vi "AO_master_DM_WFS_v1_SynModeFailure_discarded.vi"() -> ()   [LabVIEW 2018]
uses:
  <userlib>/WaveKit.lib/Controls/Image information.ctl
  <userlib>/WaveKit.lib/Controls/Image general information.ctl
  <userlib>/WaveKit.lib/Controls/Image acquisition information.ctl
  <userlib>/WaveKit.lib/Controls/Point2D.ctl
  <userlib>/WaveKit.lib/Controls/Data alignment enum.ctl
  <userlib>/WaveKit.lib/Controls/StatisticsData.ctl
  <userlib>/WaveKit.lib/Controls/Wavefront Corrector states - ONE.ctl
  <userlib>/WaveKit.lib/Classes/Camera/Camera.lvclass
  <userlib>/WaveKit.lib/Classes/CameraSet/CameraSet.lvclass
  <userlib>/WaveKit.lib/Classes/Image/Image.lvclass
  <userlib>/WaveKit.lib/Classes/Phase/Phase.lvclass
  <userlib>/WaveKit.lib/Controls/HasoSlopes.lvclass
  <userlib>/WaveKit.lib/Controls/Pupil.lvclass
  <userlib>/WaveKit.lib/Classes/WavefrontCorrector/WavefrontCorrector.lvclass
  <userlib>/WaveKit.lib/Classes/WavefrontCorrectorSet/WavefrontCorrectorSet.lvclass
  <userlib>/WaveKit.lib/Classes/HasoEngine/HasoEngine.lvclass
  <userlib>/WaveKit.lib/Controls/SlopesEngineSetup.ctl
  <userlib>/WaveKit.lib/Controls/WavefrontReconstructionMode.ctl
  <vilib>/Utility/file.llb/Read From Spreadsheet File (DBL).vi
  <vilib>/Analysis/1siggen.llb/Ramp Pattern by Delta.vi
  <userlib>/WaveKit.lib/Classes/ModalCoef/ModalCoef.lvclass
  <vilib>/Analysis/NI_AALBase.lvlib
panel:
  in  "Device Status":enum32{"DM", "WFS", "Others"}(tab)
  out "DM Actuator Values":sgl[](graph)
  out "Initial State":T1[](array[typedef])
  out "ActuatorsNumber":i32
  out "Initial Positions":sgl[](array[numeric])
  out "Final Positions":sgl[](array[numeric])
  in  "Coef Min":dbl=-0.5 min=1.0
  in  "Coef Max":dbl=0.5 min=1.0
  out "Zernike Measured":dbl[](graph)
  out "Phase statistics":T2
  out "Phase values":sgl[][](graph)=[[nan, nan, nan, nan, nan, nan, nan, nan, nan, nan, nan, nan, nan, nan, nan, nan, nan, nan, nan, nan, nan, nan, nan, nan, nan, nan, nan, nan, nan, nan, nan, nan, nan, nan, nan, nan, nan, nan, nan, nan], [nan, nan, nan, nan, nan, nan, nan, nan, nan, nan, nan, nan, nan, nan, nan, nan, nan, nan, nan, nan, nan, nan, nan, nan, nan, nan, nan, nan, nan, nan, nan, nan, nan, nan, nan, nan, nan, nan, nan, nan], [nan, nan, nan, nan, nan, nan, nan, nan, nan, nan, nan, nan, nan, nan, nan, nan, nan, nan, nan, nan, nan, nan, nan, nan, nan, nan, nan, nan, nan, nan, nan, nan, nan, nan, nan, nan, nan, nan, nan, nan], [nan, nan, nan, nan, nan, nan, nan, nan, nan, nan, nan, nan, nan, nan, nan, nan, nan, nan, nan, nan, nan, nan, nan, nan, nan, nan, nan, nan, nan, nan, nan, nan, nan, nan, nan, nan, nan, nan, nan, nan], [nan, nan, nan, nan, nan, nan, nan, nan, nan, nan, nan, nan, nan, nan, -0.14441992, nan, 0.1501734, 0.22490476, 0.2674259, 0.28415325, 0.2792031, 0.2552752, 0.21375881, 0.15405469, nan, nan, nan, nan, nan, nan, nan, nan, nan, nan, nan, nan, nan, nan, nan, nan], [nan, nan, nan, nan, nan, nan, nan, nan, nan, nan, nan, nan, nan, nan, 0.19143742, 0.2795512, 0.33646506, 0.37099743, 0.3877919, 0.3894302, 0.37774685, 0.35447162, 0.3212538, 0.27904776, 0.22675864, 0.15897867, nan, nan, nan, nan, nan, nan, nan, nan, nan, nan, nan, nan, nan, nan], [nan, nan, nan, nan, nan, nan, nan, nan, nan, nan, nan, nan, nan, 0.22618562, 0.290776, 0.33285964, 0.36044422, 0.3767934, 0.38285175, 0.37884915, 0.3652757, 0.3433441, 0.3149789, 0.28229773, 0.2464756, 0.20580466, 0.15268901, 0.06923797, nan, nan, nan, nan, nan, nan, nan, nan, nan, nan, nan, nan], [nan, nan, nan, nan, nan, nan, nan, nan, nan, nan, nan, nan, 0.19992779, 0.24616541, 0.27565512, 0.29675642, 0.31222007, 0.32191983, 0.32467726, 0.31943765, 0.30597392, 0.2852214, 0.25927368, 0.2309889, 0.20308714, 0.17653626, 0.14795627, 0.10568966, 0.024115691, nan, nan, nan, nan, nan, nan, nan, nan, nan, nan, nan], [nan, nan, nan, nan, nan, nan, nan, nan, nan, nan, nan, 0.14862825, 0.18219855, 0.20114602, 0.21551609, 0.22862102, 0.24014233, 0.24817906, 0.2505626, 0.24567793, 0.23295718, 0.21313797, 0.18829979, 0.16161954, 0.1367108, 0.11633411, 0.10019377, 0.081457645, 0.04156301, -0.057204023, nan, nan, nan, nan, nan, nan, nan, nan, nan, nan], [nan, nan, nan, nan, nan, nan, nan, nan, nan, nan, 0.08899155, 0.117771566, 0.12948777, 0.13732892, 0.14631097, 0.15688494, 0.16728252, 0.17497937, 0.17758016, 0.17335457, 0.16157834, 0.14275661, 0.11873307, 0.09261118, 0.06834036, 0.04974218, 0.038678437, 0.031985473, 0.016725859, -0.03676957, nan, nan, nan, nan, nan, nan, nan, nan, nan, nan], [nan, nan, nan, nan, nan, nan, nan, nan, nan, nan, 0.058377307, 0.069048055, 0.0725615, 0.07683456, 0.0840318, 0.09335055, 0.10271386, 0.1097376, 0.11226265, 0.10867052, 0.09812171, 0.08078306, 0.058033932, 0.032565817, 0.008214329, -0.010712444, -0.020921554, -0.022825297, -0.02489755, -0.05023362, -0.14592764, nan, nan, nan, nan, nan, nan, nan, nan, nan], [nan, nan, nan, nan, nan, nan, nan, nan, nan, -0.0018393314, 0.018310271, 0.023098737, 0.024714457, 0.027986258, 0.033823933, 0.041292578, 0.048749834, 0.054400377, 0.056548227, 0.05374936, 0.04499338, 0.029967438, 0.009379062, -0.014759185, -0.03905803, -0.059140373, -0.070816256, -0.0724436, -0.06894927, -0.07806298, -0.1393881, nan, nan, nan, nan, nan, nan, nan, nan, nan], [nan, nan, nan, nan, nan, nan, nan, nan, nan, -0.03322208, -0.017045017, -0.0123043535, -0.010394985, -0.007970343, -0.0042642877, 0.0003761826, 0.005164365, 0.009095938, 0.010986101, 0.009512841, 0.0033822758, -0.008344227, -0.02579559, -0.047820807, -0.071688615, -0.09321856, -0.107681155, -0.11187886, -0.10789668, -0.10908524, -0.14891545, -0.29341945, nan, nan, nan, nan, nan, nan, nan, nan], [nan, nan, nan, nan, nan, nan, nan, nan, nan, nan, -0.043187555, -0.03622458, -0.033755217, -0.03278728, -0.03198469, -0.030707732, -0.028716512, -0.026208155, -0.023933899, -0.023217455, -0.025771504, -0.03328519, -0.04682974, -0.06620631, -0.08943447, -0.1126552, -0.13079928, -0.13944486, -0.13836564, -0.13734597, -0.16491348, -0.2807172, nan, nan, nan, nan, nan, nan, nan, nan], [nan, nan, nan, nan, nan, nan, nan, nan, -0.13038255, -0.08328184, -0.060542934, -0.050779276, -0.048053104, -0.048984695, -0.05126809, -0.053124577, -0.05330209, -0.051303368, -0.04760214, -0.04368073, -0.041799206, -0.04448101, -0.05377527, -0.07043236, -0.09320336, -0.118551016, -0.14113419, -0.15550357, -0.15952203, -0.16009864, -0.18189941, -0.27977645, nan, nan, nan, nan, nan, nan, nan, nan], [nan, nan, nan, nan, nan, nan, nan, nan, -0.15416794, -0.09987456, -0.07151361, -0.05893044, -0.056102008, -0.058817875, -0.063637674, -0.067669004, -0.06878706, -0.06599128, -0.059670344, -0.051622536, -0.044753395, -0.042448726, -0.04769562, -0.062100213, -0.08502676, -0.11315687, -0.14084403, -0.16171429, -0.1720384, -0.17647736, -0.19687745, -0.284868, -0.53908885, -1.12795, nan, nan, nan, nan, nan, nan], [nan, nan, nan, nan, nan, nan, nan, nan, -0.17633308, -0.1131372, -0.07876157, -0.06330658, -0.060116876, -0.063924976, -0.07015394, -0.07493687, -0.07548633, -0.07052183, -0.060539607, -0.047784284, -0.035856243, -0.028966732, -0.030924596, -0.044017438, -0.06802279, -0.099662215, -0.13288532, -0.16044727, -0.17731819, -0.18653797, -0.20820689, -0.29237592, -0.5366785, nan, nan, nan, nan, nan, nan, nan], [nan, nan, nan, nan, nan, nan, nan, nan, -0.19826387, -0.12505035, -0.08430402, -0.06564974, -0.061443567, -0.06527472, -0.07152294, -0.07554153, -0.07411167, -0.0658889, -0.05163869, -0.034133032, -0.017655006, -0.0071354215, -0.007018423, -0.020031396, -0.046107426, -0.08178567, -0.12048963, -0.15415914, -0.17678727, -0.19048853, -0.21480094, -0.2999987, -0.54526997, nan, nan, nan, nan, nan, nan, nan], [nan, nan, nan, nan, nan, nan, nan, nan, -0.2214154, -0.13693352, -0.08914254, -0.06661926, -0.06048554, -0.06317037, -0.0681367, -0.07015528, -0.065784656, -0.053790003, -0.035310905, -0.013662348, 0.0062713036, 0.01901285, 0.01972933, 0.005542416, -0.023349542, -0.06307545, -0.10643376, -0.14466219, -0.17119798, -0.18806857, -0.21562657, -0.30642, -0.5640642, nan, nan, nan, nan, nan, nan, nan], [nan, nan, nan, nan, nan, nan, nan, nan, -0.24718054, -0.14940841, -0.093277775, -0.0658183, -0.056708053, -0.05720259, -0.059951056, -0.05929426, -0.051715773, -0.036192447, -0.014265999, 0.010266874, 0.032073133, 0.04536258, 0.04520398, 0.028878966, -0.0030008797, -0.045963787, -0.092160165, -0.13235793, -0.16002774, -0.17817038, -0.20961209, -0.31157303, -0.5953845, nan, nan, nan, nan, nan, nan, nan], [nan, nan, nan, nan, nan, nan, nan, nan, -0.27748746, -0.16290864, -0.09610232, -0.062047683, -0.048735943, -0.04617936, -0.046241976, -0.042900223, -0.03261665, -0.014586102, 0.009311387, 0.03494107, 0.05674191, 0.068891875, 0.0666744, 0.04783368, 0.0136316735, -0.030755527, -0.0769404, -0.115639456, -0.14119013, -0.15893419, -0.19620675, -0.31774768, nan, nan, nan, nan, nan, nan, nan, nan], [nan, nan, nan, nan, nan, nan, nan, nan, -0.31623095, -0.17884897, -0.09729818, -0.0539262, -0.03469713, -0.028198741, -0.025418447, -0.019910373, -0.008048305, 0.010862423, 0.034768496, 0.05942371, 0.07931873, 0.0889112, 0.08400761, 0.06307276, 0.028166434, -0.014867521, -0.057410896, -0.09080534, -0.111413695, -0.12868427, -0.17697167, -0.3319423, nan, nan, nan, nan, nan, nan, nan, nan], [nan, nan, nan, nan, nan, nan, nan, nan, nan, -0.20170604, -0.09850275, -0.0411539, -0.0131010795, -0.0011654077, 0.0047943285, 0.01185911, 0.023955166, 0.041901454, 0.06374147, 0.08542206, 0.1018104, 0.10796184, 0.10047772, 0.0787158, 0.04554086, 0.007227666, -0.027947046, -0.052963093, -0.06777905, -0.08820889, -0.15871821, nan, nan, nan, nan, nan, nan, nan, nan, nan], [nan, nan, nan, nan, nan, nan, nan, nan, nan, -0.24239759, -0.10614249, -0.026831074, 0.015322472, 0.03581071, 0.046350636, 0.05505173, 0.06651187, 0.08204405, 0.10016226, 0.11737824, 0.12928592, 0.13183476, 0.12261822, 0.10192663, 0.073240966, 0.042765103, 0.017522467, 0.0014635092, -0.0110412, -0.045025453, -0.15884721, nan, nan, nan, nan, nan, nan, nan, nan, nan], [nan, nan, nan, nan, nan, nan, nan, nan, nan, nan, -0.13597216, -0.021381527, 0.04426403, 0.07956008, 0.09847209, 0.110732496, 0.122154154, 0.13505057, 0.14887714, 0.16113368, 0.16849175, 0.16803522, 0.1584293, 0.14075197, 0.118653886, 0.09743117, 0.0815231, 0.06987105, 0.048498146, -0.020404778, nan, nan, nan, nan, nan, nan, nan, nan, nan, nan], [nan, nan, nan, nan, nan, nan, nan, nan, nan, nan, nan, -0.04876471, 0.05625415, 0.117832564, 0.15310521, 0.17423762, 0.18897903, 0.20128381, 0.21210447, 0.22038196, 0.22418612, 0.221881, 0.21311647, 0.19937092, 0.1836943, 0.16922635, 0.15598845, 0.13537171, 0.081669986, nan, nan, nan, nan, nan, nan, nan, nan, nan, nan, nan], [nan, nan, nan, nan, nan, nan, nan, nan, nan, nan, nan, nan, 0.014031529, 0.121263236, 0.18738765, 0.22803904, 0.25380248, 0.2710389, 0.28282017, 0.2899857, 0.29225817, 0.2892868, 0.28139976, 0.26978248, 0.25571787, 0.23844866, 0.21115, 0.15442081, nan, nan, nan, nan, nan, nan, nan, nan, nan, nan, nan, nan], [nan, nan, nan, nan, nan, nan, nan, nan, nan, nan, nan, nan, nan, nan, 0.15212902, 0.2306162, 0.28129596, 0.31381333, 0.33402625, 0.3450995, 0.34855807, 0.34515002, 0.33529556, 0.31882071, 0.29360068, 0.25266168, nan, nan, nan, nan, nan, nan, nan, nan, nan, nan, nan, nan, nan, nan], [nan, nan, nan, nan, nan, nan, nan, nan, nan, nan, nan, nan, nan, nan, nan, nan, 0.1979487, 0.2623494, 0.30271748, 0.32490522, 0.33223343, 0.3261181, 0.30614072, 0.26925305, nan, nan, nan, nan, nan, nan, nan, nan, nan, nan, nan, nan, nan, nan, nan, nan], [nan, nan, nan, nan, nan, nan, nan, nan, nan, nan, nan, nan, nan, nan, nan, nan, nan, nan, nan, nan, nan, nan, nan, nan, nan, nan, nan, nan, nan, nan, nan, nan, nan, nan, nan, nan, nan, nan, nan, nan], [nan, nan, nan, nan, nan, nan, nan, nan, nan, nan, nan, nan, nan, nan, nan, nan, nan, nan, nan, nan, nan, nan, nan, nan, nan, nan, nan, nan, nan, nan, nan, nan, nan, nan, nan, nan, nan, nan, nan, nan], [nan, nan, nan, nan, nan, nan, nan, nan, nan, nan, nan, nan, nan, nan, nan, nan, nan, nan, nan, nan, nan, nan, nan, nan, nan, nan, nan, nan, nan, nan, nan, nan, nan, nan, nan, nan, nan, nan, nan, nan]] caption="Wavefront"
  out "HASO intensity":u32[][](graph)
  out "Current error":errorcluster
  out "Output path":path=path "D:/Data"
  in  "Current status":string="Test1"
  out "HASO ready":bool
  in  "Live Wavefront":bool
  in  "Update DM":bool
  in  "Tab Control":T3(tab)
  in  "Initial haso file":path=path "D:/SystemAlignment/system_aberration_residual_20211023_2.has"
  in  "interaction matrix file":path=path "D:/SystemAlignment/IM_20211023_0p5x2_500nm_2.aomi"
  in  "DM configuration file":path=path "C:/Program Files (x86)/Imagine Optic/Configuration Files/WaveFrontCorrector_mirao52-e_0326.dat"
  in  "Haso configuration file":path=path "C:/Program Files (x86)/Imagine Optic/Configuration Files/HASO3_first_7364.dat"
  in  "Coef value":dbl=0.5 min=1.0
  in  "Idx end":u32=20 min=1
  in  "Idx start":u32=1 min=1
  in  "Subfolder":string="Test1"
  in  "Folder Name":string="Test"
  in  "Record Response":bool
  in  "Net Rp":bool
  in  "Input type":T4(ring)=enum."Zernike Coef"
  in  "Additional Command":bool=TRUE
  in  "Offset command file":path=path "D:/SystemAlignment/system_aberration_20211103.dat"
  in  "Initial offset":bool=TRUE
  in  "Additional file":path=path "D:/SystemAlignment/system_aberration_20191029.dat"
  out "Zern coef out":sgl[](array[numeric])
  out "Zern index out":i32[](array[numeric])
  in  "Zern index in":i32[](array[numeric])
  in  "Zern coef in":sgl[](array[numeric])
  in  "idxType":enum16{"Wyant", "ANSI"}(ring)
  in  "Filter":u8[](array[numeric])
  out "exposure_duration_us (get)":u32
  in  "exposure_duration_s (set)":dbl=1.0 min=1.0
  out "nb_images (get)":u32=10
  in  "nb_images (set)":u32=1 min=1
  in  "Save File":bool
  in  "File Base Name":string="Test"
  in  "Main Path":path=path "D:/Data"
  in  "Record Batch":bool
  out "Acquisition information":T5={"Image general information"={"Camera serial number"="", "Smearing removed"=FALSE, "Background image removed"=FALSE, "Time Stamp"=timestamp(0 s since 1904-01-01), "Comment"="", "Camera_MAX_Level"=0}, "Acquisition information"={"Exposure duration (us)"=0, "Exposure duration specified (us)"=0, "Gain"=0.0, "Number of summed images"=0, "Trigger type"=""}, "Number of pixels"={"X"=0, "Y"=0}, "Number of bits"=enum."16"}
  in  "Init":bool
  in  "Reset error":bool
  in  "Exit":bool
  in  "Stop HASO":bool
  in  "Start HASO":bool
  # "AO_master_DM_WFS_v1.vi: (last update:  discarded 20211214 )\nControl deformable mirror and wavefront sensor, check DM response be WFS \n1, re-orgnize panel/interface: tap for settings, tab for display and indicators\n2, change camera asynchronous mode to synchronous mode (??does not work)\n3, add control to flip mirror. (laser shutter and stage ???)\n4, Make it more efficient and robust to errors\na) DM ocuppied due to last unnormal exit; b) wavefront measure error: no laser, wrong slopes;"
  # "syn mode does not work when exp time > 0.1s??"
  # "um"
  # "HASO Parameters"
  # "Check DM Response"
  # "Need to turn OFF live wavefront"
  # "Batch range"
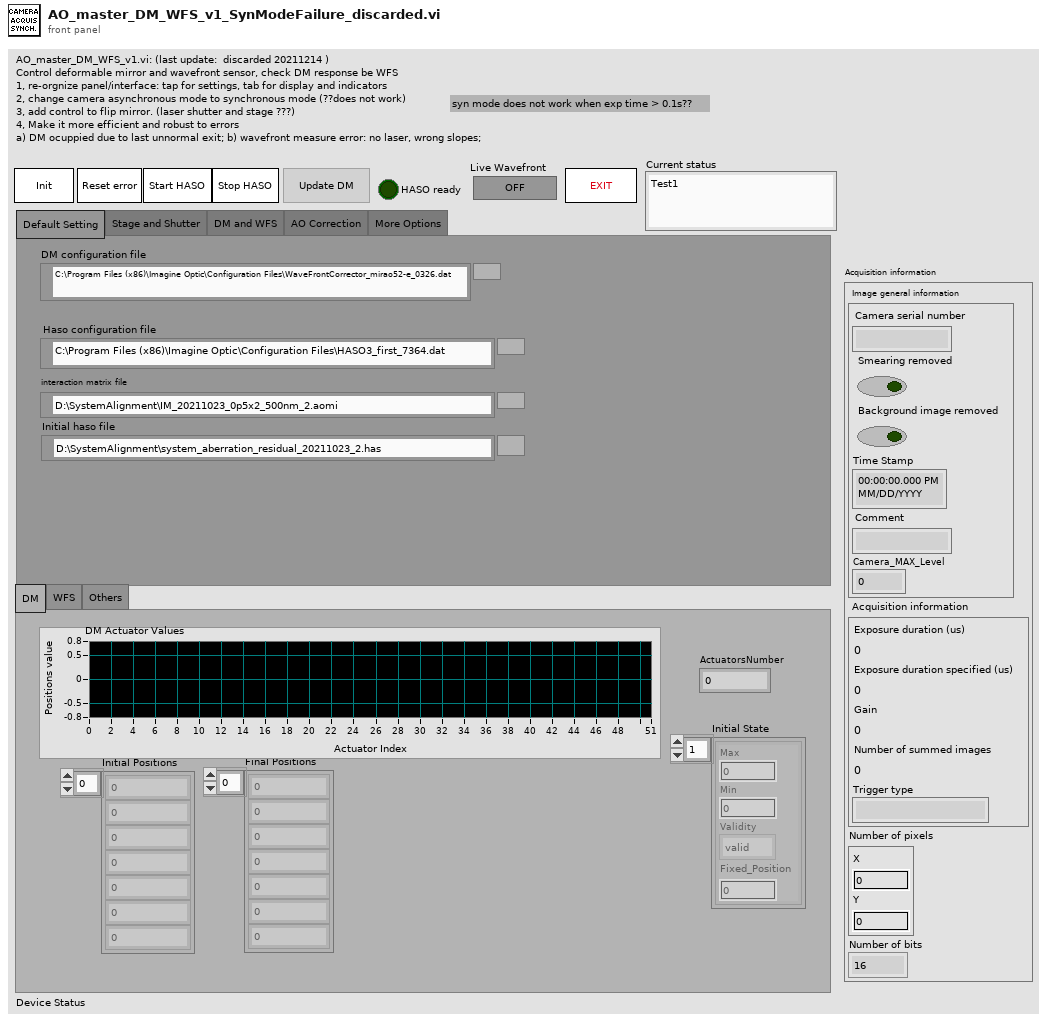
[diagram p1: front panel]
types:
  T1 = typedef "Wavefront Corrector states - ONE.ctl" = cluster{"Max":sgl, "Min":sgl, "Validity":enum16{"valid", "fixed", "invalid"}, "Fixed_Position":sgl}
  T2 = typedef "StatisticsData.ctl" = cluster{"PV":sgl, "RMS":dbl, "Max":sgl, "Min":sgl}
  T3 = enum32{"Default Setting", "Stage and Shutter", "DM and WFS", "AO Correction", "More Options"}
  T4 = enum16{"Zero Input", "Command File", "Zernike Coef", "Zernike File"}
  T5 = typedef "Image information.ctl" = cluster{"Image general information":T6, "Acquisition information":T7, "Number of pixels":T8, "Number of bits":T9}
  T6 = typedef "Image general information.ctl" = cluster{"Camera serial number":string, "Smearing removed":bool, "Background image removed":bool, "Time Stamp":timestamp, "Comment":string, "Camera_MAX_Level":i32}
  T7 = typedef "Image acquisition information.ctl" = cluster{"Exposure duration (us)":i32, "Exposure duration specified (us)":i32, "Gain":sgl, "Number of summed images":i32, "Trigger type":string}
  T8 = typedef "Point2D.ctl" = cluster{"X":u32, "Y":u32}
  T9 = typedef "Data alignment enum.ctl" = enum16{"8", "16", "32"}
  T10 = typedef "SlopesEngineSetup.ctl" = cluster{"Start sub-aperture":T8, "Pupil average":dbl}
  T11 = typedef "CameraSpecifications.ctl" = cluster{"Grabber name":string, "Camera name":string, "Camera sn":string, "Pixels_um":T12, "Maximum level":u32, "Data alignment":T9, "Is signed":bool, "Acquisition start":T8, "Acquisition length":T8, "MaxFrameRate_Hz":sgl, "Chip type":enum16{"Progressive scan", "Frame transfert"}}
  T12 = typedef "General dimensions definition.ctl" = cluster{"Size":T8, "Step":T13}
  T13 = typedef "Point2Df.ctl" = cluster{"X":sgl, "Y":sgl}
  T14 = typedef "Wavefront Corrector Position.ctl" = sgl[]
  T15 = typedef "WavefrontReconstructionMode.ctl" = enum16{"None", "Modal_Legendre", "Modal_Zernike", "Zonal", "Modal_Zonal_Zernike", "Modal_Zonal_Legendre"}
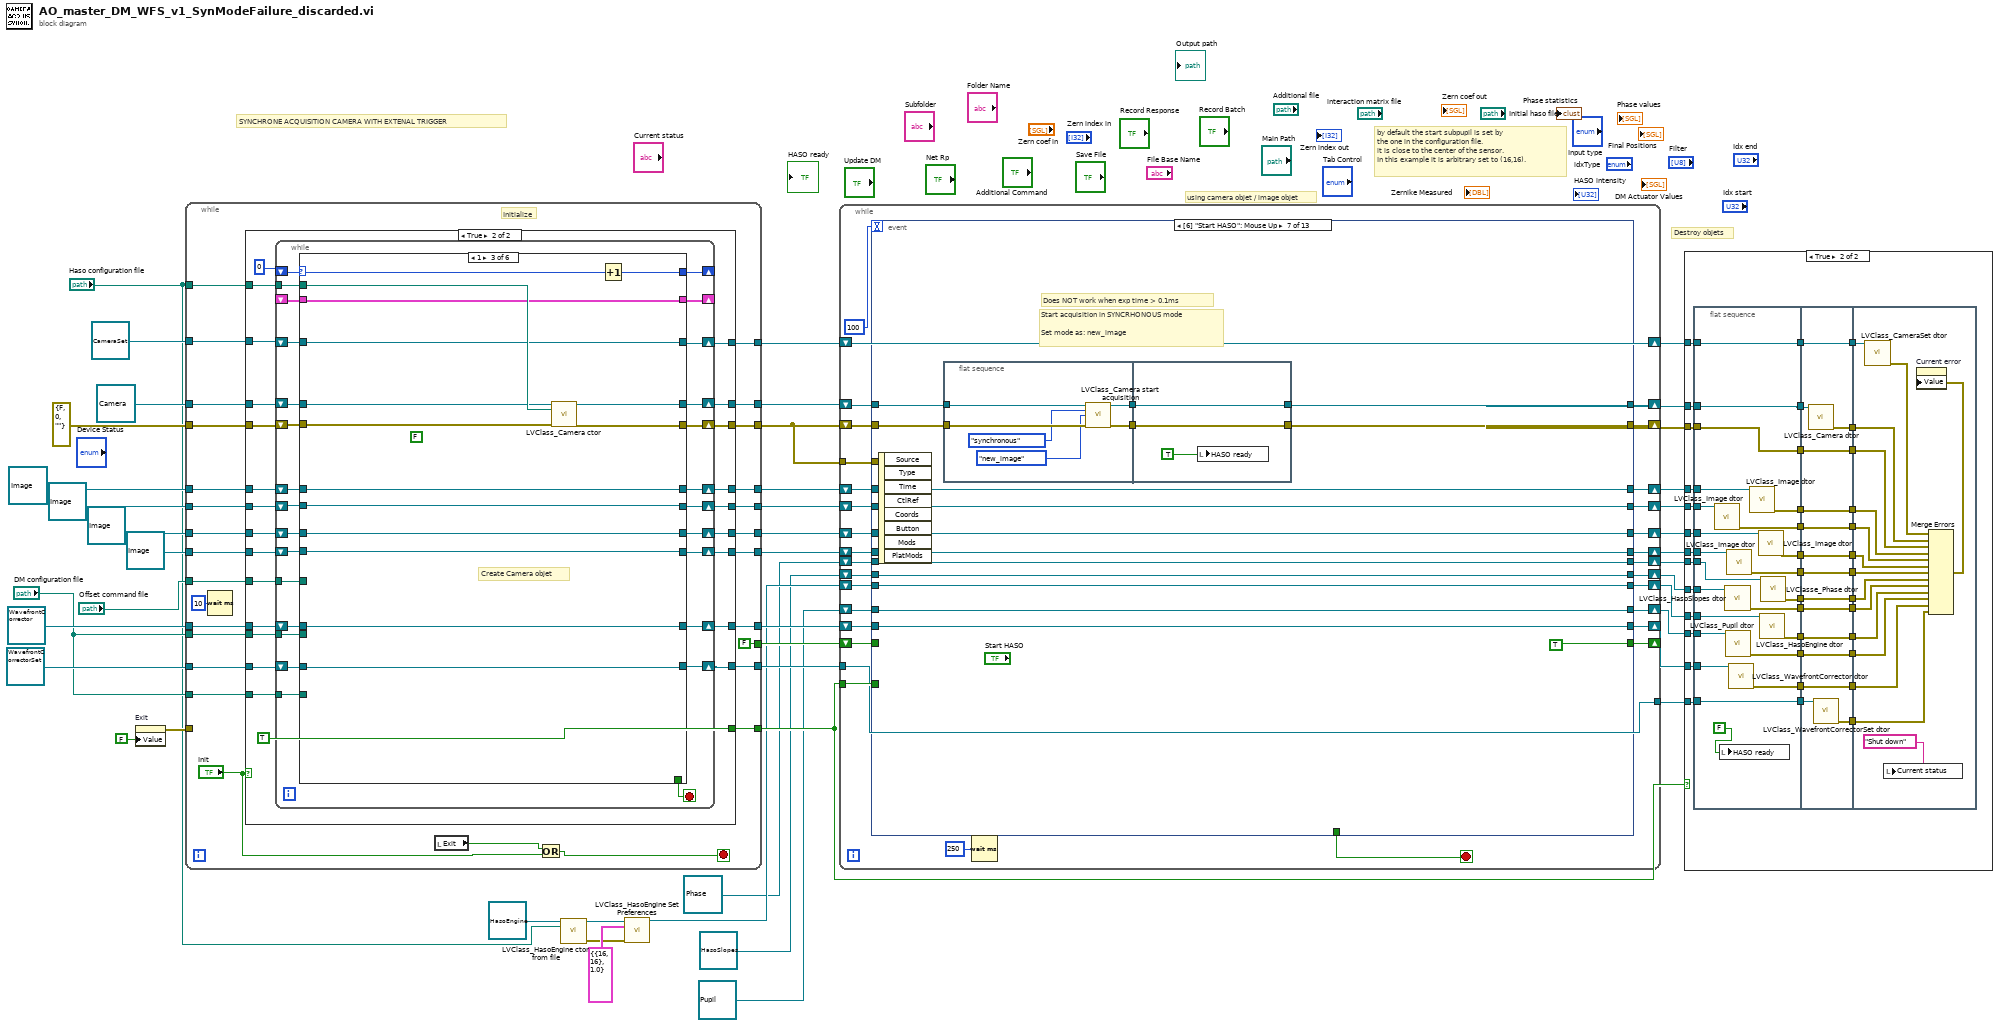
[diagram p0: block diagram]
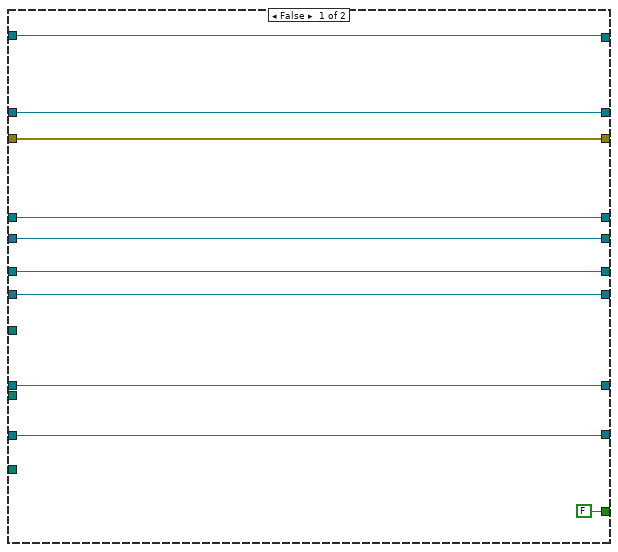
[diagram p3: hidden frame]
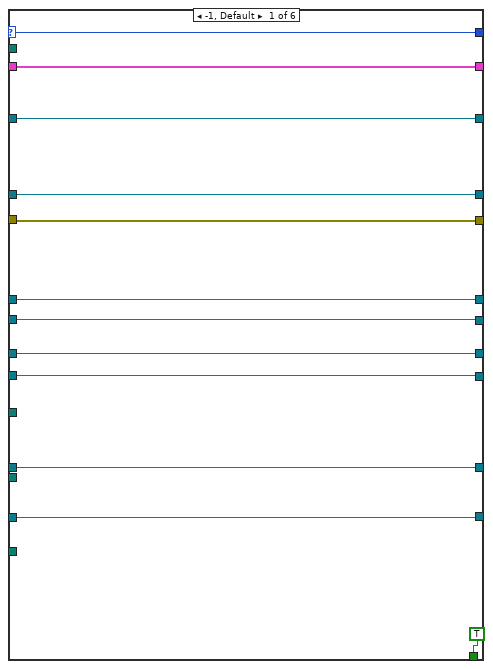
[diagram p4: hidden frame]
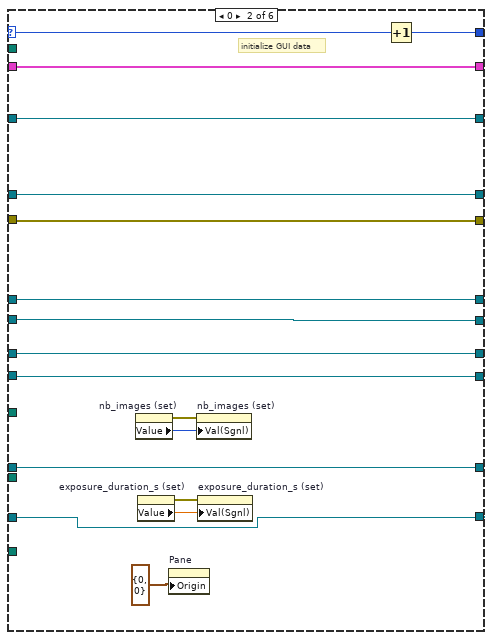
[diagram p5: hidden frame]
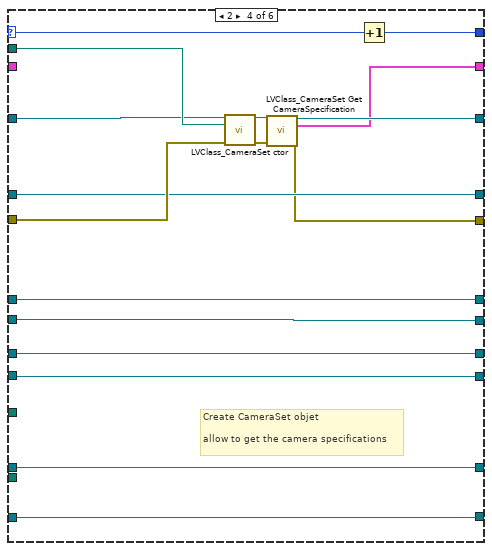
[diagram p6: hidden frame]
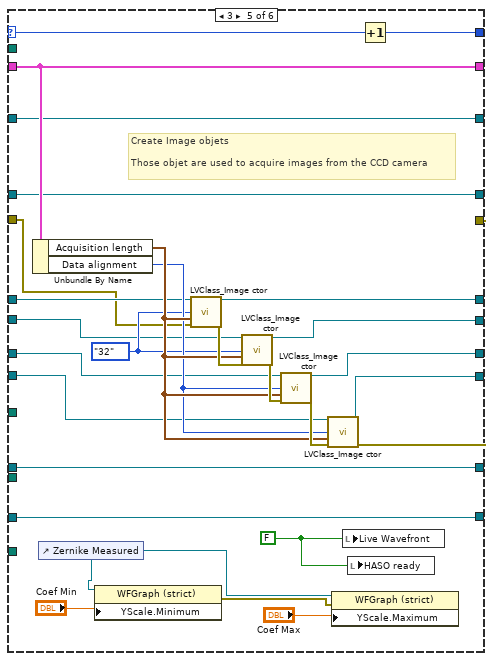
[diagram p7: hidden frame]
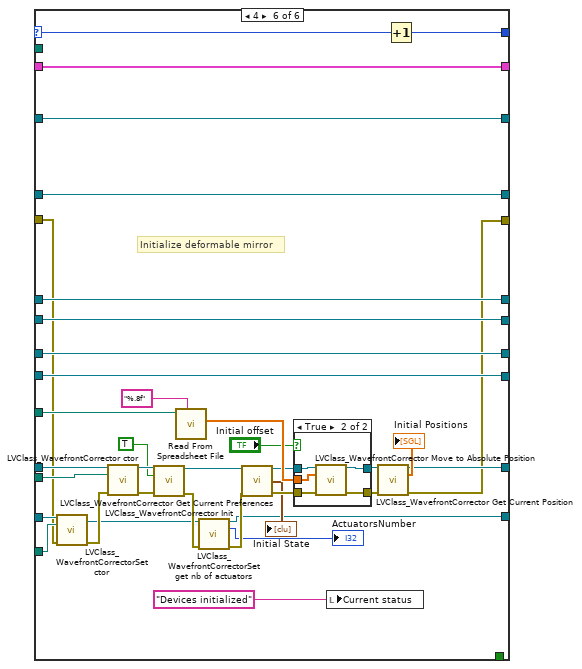
[diagram p8: hidden frame]
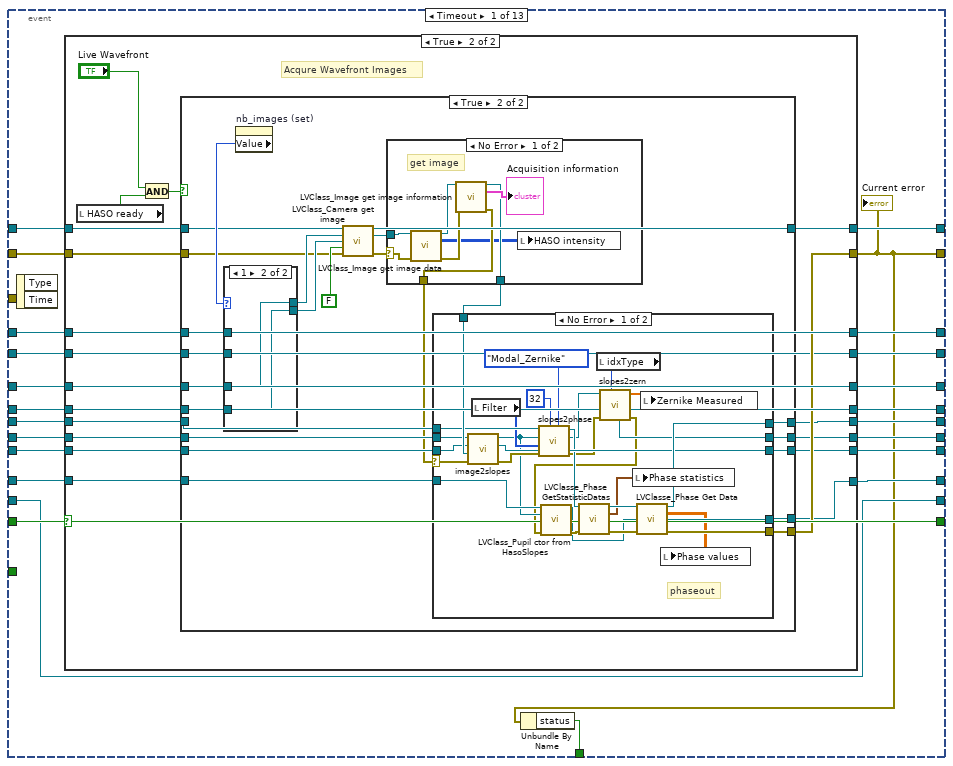
[diagram p10: hidden frame]
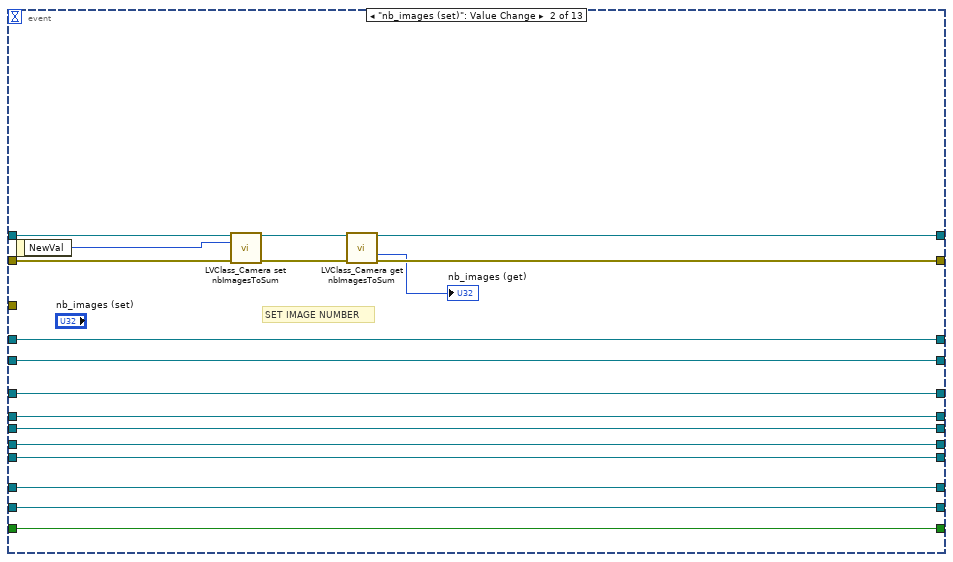
[diagram p16: hidden frame]
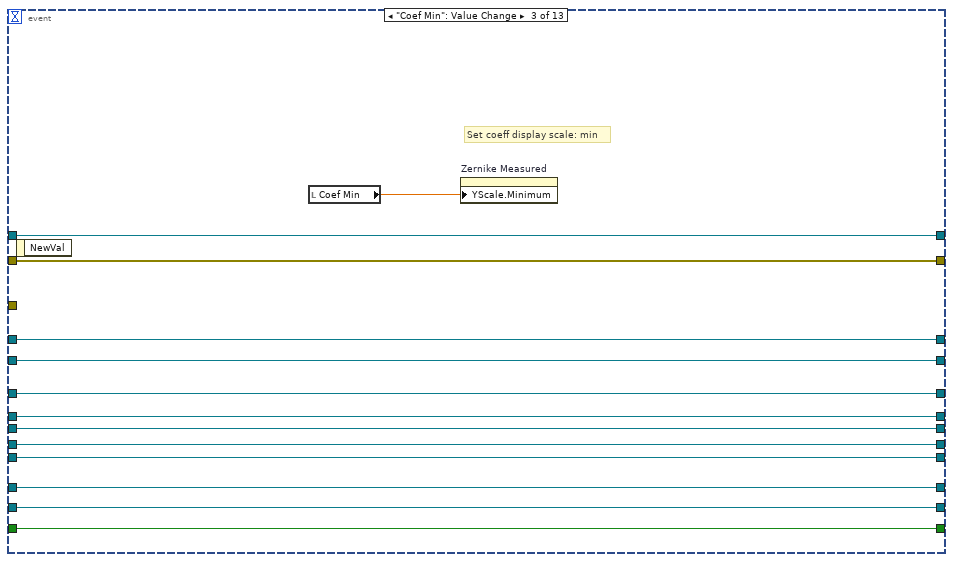
[diagram p17: hidden frame]
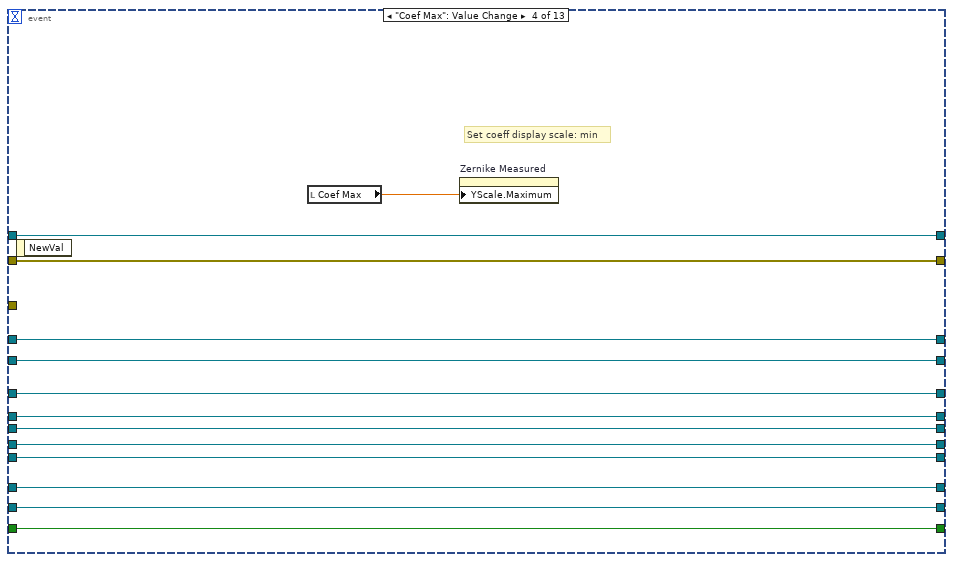
[diagram p18: hidden frame]
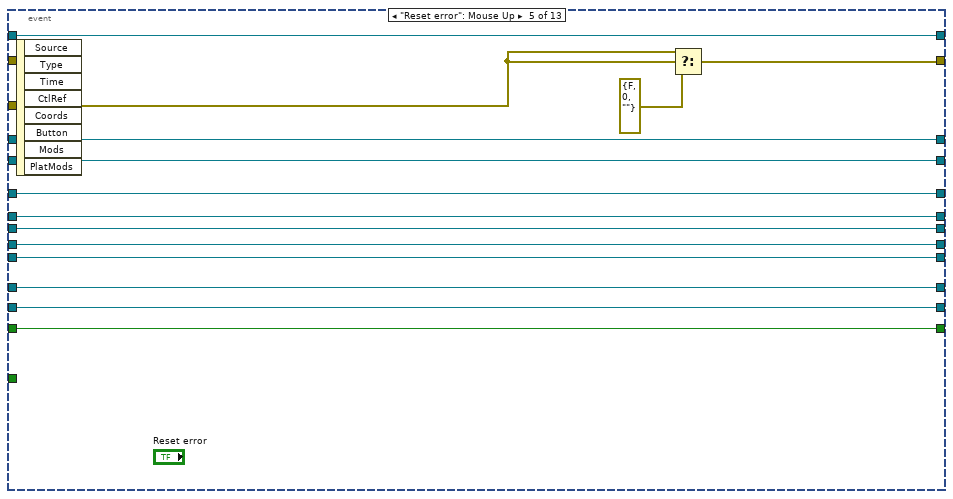
[diagram p19: hidden frame]
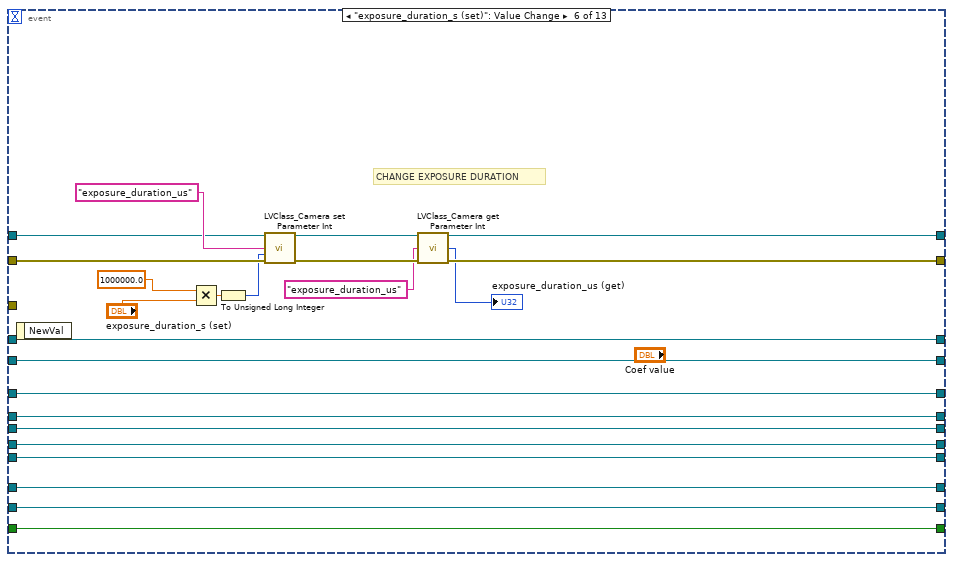
[diagram p20: hidden frame]
diagram:
  # "by default the start subpupil is set by \nthe one in the configuration file. \nit is close to the center of the sensor.\nIn this example it is arbitrary set to (16,16)."
  # "Destroy objets"
  # "using camera objet / image objet"
  # "SYNCHRONE ACQUISITION CAMERA WITH EXTENAL TRIGGER"
  n1 = property on="Exit" class="Bool (strict)"("Value"=FALSE ("Exit")) -> (error out=w22:errorcluster)  [unwired: 2 in, 1 out]
  n2 = while {
    tunnel: [FALSE] -> w39
    tunnel: [w73] -> w38
    tunnel: [w72] -> w37
    tunnel: [w71] -> w36
    tunnel: [w70] -> w35
    tunnel: [w69] -> w34
    tunnel: [w68] -> w33
    tunnel: refnum<class "Camera.lvclass"> refnum ("Camera.lvclass") -> [w67]
    tunnel: refnum<class "CameraSet.lvclass"> refnum ("CameraSet.lvclass") -> [w66]
    tunnel: refnum<class "Image.lvclass"> refnum ("Image in") -> [w65]
    tunnel: refnum<class "Image.lvclass"> refnum ("Image in") -> [w64]
    tunnel: refnum<class "Image.lvclass"> refnum ("Image in") -> [w63]
    tunnel: refnum<class "Image.lvclass"> refnum ("Image in") -> [w62]
    tunnel: errorcluster {"status"=FALSE, "code"=0, "source"=""} ("error out") -> [w61]
    tunnel: [w60] -> w25
    tunnel: [w58] -> w24
    tunnel: w22 -> [_]
    tunnel: "Haso configuration file" -> [w54]
    tunnel: "Offset command file" -> [w53]
    tunnel: refnum<class "WavefrontCorrectorSet.lvclass"> refnum ("WavefrontCorrectorSet in") -> [w52]
    tunnel: "DM configuration file" -> [w51]
    tunnel: refnum<class "WavefrontCorrector.lvclass"> refnum ("WavefrontCorrector in") -> [w50]
    tunnel: "DM configuration file" -> [w49]
    tunnel: [w48] -> w17
    tunnel: [w47] -> w16
    stop <- w55 stop-if-true
    # "Initialize"
    n3 = Wait (ms)(milliseconds to wait=u32 10) -> ()  [unwired: 1 out]
    n4 = case shown="True" "Init" {
      tunnel: [w84 w108] -> w73
      tunnel: [w83 w107] -> w72
      tunnel: [w81 w106] -> w71
      tunnel: [w80 w105] -> w70
      tunnel: [w79 w104] -> w69
      tunnel: [w78 w103] -> w68
      tunnel: w67 -> [w84 w102]
      tunnel: w66 -> [w83 w100]
      tunnel: w65 -> [w81 w99]
      tunnel: w64 -> [w80 w98]
      tunnel: w63 -> [w79 w97]
      tunnel: w62 -> [w78 w96]
      tunnel: w61 -> [w82 w95]
      tunnel: [w82 w94] -> w60
      tunnel: [FALSE TRUE] -> w58
      tunnel: w54 -> [_ w92]
      tunnel: w53 -> [_ w91]
      tunnel: w52 -> [w75 w85]
      tunnel: w51 -> [_ w90]
      tunnel: w50 -> [w76 w86]
      tunnel: w49 -> [_ w89]
      tunnel: [w76 w88] -> w48
      tunnel: [w75 w87] -> w47
      frame False {
      }
      frame True {
        n5 = while {
          tunnel: w92 -> [w133]
          shift-right: [w135] -> w108
          shift-left: w102 -> [w127]
          shift-right: [w117] -> _
          shift-left: 0 -> [w116]
          shift-right: [w134] -> w107
          shift-left: w100 -> [w126]
          shift-right: [w125] -> _
          shift-left: _ -> [w123]
          shift-right: [w132] -> w106
          shift-left: w99 -> [w124]
          shift-right: [w131] -> w105
          shift-left: w98 -> [w122]
          shift-right: [w130] -> w104
          shift-left: w97 -> [w120]
          shift-right: [w129] -> w103
          shift-left: w96 -> [w121]
          shift-right: [w128] -> w94
          shift-left: w95 -> [w118]
          tunnel: w91 -> [w115]
          tunnel: w90 -> [w114]
          tunnel: w89 -> [w113]
          shift-right: [w112] -> w88
          shift-left: w86 -> [w110]
          shift-right: [w111] -> w87
          shift-left: w85 -> [w109]
          stop <- w119 stop-if-true
          n6 = case shown="1" w116 {
            tunnel: [w147 w151 w179 w189 w211 w261] -> w135
            tunnel: w133 -> [_ _ w178 w193 _ _]
            tunnel: [w146 w155 w176 w194 w212 w260] -> w134
            tunnel: [w139 w156 w170 w184 w218 w255] -> w132
            tunnel: [w140 w157 w171 w185 w217 w256] -> w131
            tunnel: [w141 w158 w172 w186 w216 w257] -> w130
            tunnel: [w142 w159 w173 w187 w215 w258] -> w129
            tunnel: [w143 w150 w175 w188 w214 w229] -> w128
            selector: w116 -> [w138 w153 w168 w183 w206 w227]
            tunnel: w127 -> [w147 w151 w177 w189 w211 w261]
            tunnel: w126 -> [w146 w155 w176 w192 w212 w260]
            tunnel: [w144 w152 w174 w191 w213 w259] -> w125
            tunnel: w124 -> [w139 w156 w170 w184 w210 w255]
            tunnel: w123 -> [w144 w152 w174 _ w213 w259]
            tunnel: w122 -> [w140 w157 w171 w185 w209 w256]
            tunnel: w121 -> [w142 w159 w173 w187 w208 w258]
            tunnel: w120 -> [w141 w158 w172 w186 w207 w257]
            tunnel: [TRUE _ _ _ _ _] -> w119
            tunnel: w118 -> [w143 w150 w167 w190 w204 w230]
            tunnel: [w138 w154 w169 w182 w205 w226] -> w117
            tunnel: w115 -> [_ _ _ _ _ w237]
            tunnel: w109 -> [w136 w148 w165 w180 w202 w235]
            tunnel: w114 -> [_ _ _ _ _ w234]
            tunnel: w110 -> [w137 w149 w166 w181 w203 w233]
            tunnel: w113 -> [_ _ _ _ _ w232]
            tunnel: [w137 w149 w166 w181 w203 w231] -> w112
            tunnel: [w136 w148 w165 w180 w202 w228] -> w111
            frame -1, Default {
            }
            frame 0 {
              # "initialize GUI data"
              n7 = property on="nb_images (set)" class="DigNum (strict)"() -> (error out=w164:errorcluster, "Value"=w163:u32)  [unwired: 2 in, 1 out]
              n8 = property on="exposure_duration_s (set)" class="DigNum (strict)"() -> (error out=w160:errorcluster, "Value"=w162:dbl)  [unwired: 2 in, 1 out]
              n9 = property on="Pane" class="Pane"("Origin"=cluster{"Horizontal":i16, "Vertical":i16} {"Horizontal"=0, "Vertical"=0} ("Front Panel Window:Origin")) -> ()  [unwired: 2 in, 2 out]
              n10 = property on="nb_images (set)" class="DigNum (strict)"(error in=w164, "Val(Sgnl)"=w163) -> ()  [unwired: 1 in, 2 out]
              n11 = property on="exposure_duration_s (set)" class="DigNum (strict)"(error in=w160, "Val(Sgnl)"=w162) -> ()  [unwired: 1 in, 2 out]
              n12 = Increment(x=w153) -> (x+1=w154:i32)
            }
            frame 1 {
              (unwired) FALSE ("Acq required")
              # "Create Camera objet"
              n13 = call <userlib>:"LVClass_Camera ctor.vi"("Camera"=w177, "Configuration file path"=w178, "error in (no error)"=w167) -> ("Camera (new)"=w179:refnum<class "Camera.lvclass">, "error out"=w175:errorcluster)  [unwired: 11 in]
              n14 = Increment(x=w168) -> (x+1=w169:i32)
            }
            frame 2 {
              # "Create CameraSet objet\n\nallow to get the camera specifications"
              n15 = call <userlib>:"LVClass_CameraSet ctor.vi"("CameraSet.lvclass"=w192, "Configuration file path"=w193, "error in (no error)"=w190) -> ("CameraSet.lvclass"=w196:refnum<class "CameraSet.lvclass">, "error out"=w195:errorcluster)  [unwired: 11 in]
              n16 = call <userlib>:"LVClass_CameraSet Get CameraSpecification.vi"("CameraSet.lvclass"=w196, "error in (no error)"=w195) -> ("CameraSet.lvclass"=w194:refnum<class "CameraSet.lvclass">, "Camera Config"=w191:T11, "error out"=w188:errorcluster)  [unwired: 11 in]
              n17 = Increment(x=w183) -> (x+1=w182:i32)
            }
            frame 3 {
              w201 = FALSE
              w219 = Data_alignment_enum."32" ("Data alignment")
              # "Create Image objets\n\nThose objet are used to acquire images from the CCD camera"
              n18 = Unbundle By Name(w213) -> ("Acquisition length"=w221:T8, "Data alignment"=w220:T9)
              n19 = control-ref of="Zernike Measured"() -> (w198:refnum<vi>)
              n20 = property on="Property Node" class="WFGraph (strict)"(reference=w198, "YScale.Minimum"="Coef Min") -> (error out=w197:errorcluster)  [unwired: 1 in, 1 out]
              n21 = call <userlib>:"LVClass_Image ctor.vi"("Image in"=w210, "Data alignment"=w219, "Size"=w221, "error in (no error)"=w204) -> ("Image out"=w218:refnum<class "Image.lvclass">, "error out"=w222:errorcluster)  [unwired: 10 in]
              n22 = call <userlib>:"LVClass_Image ctor.vi"("Image in"=w209, "Data alignment"=w219, "Size"=w221, "error in (no error)"=w222) -> ("Image out"=w217:refnum<class "Image.lvclass">, "error out"=w223:errorcluster)  [unwired: 10 in]
              n23 = call <userlib>:"LVClass_Image ctor.vi"("Image in"=w207, "Data alignment"=w220, "Size"=w221, "error in (no error)"=w223) -> ("Image out"=w216:refnum<class "Image.lvclass">, "error out"=w224:errorcluster)  [unwired: 10 in]
              n24 = call <userlib>:"LVClass_Image ctor.vi"("Image in"=w208, "Data alignment"=w220, "Size"=w221, "error in (no error)"=w224) -> ("Image out"=w215:refnum<class "Image.lvclass">, "error out"=w214:errorcluster)  [unwired: 10 in]
              n25 = property on="Property Node" class="WFGraph (strict)"(reference=w198, error in=w197, "YScale.Maximum"="Coef Max") -> ()  [unwired: 2 out]
              n26 = local write "Live Wavefront"(w201) -> ()
              n27 = local write "HASO ready"(w201) -> ()
              n28 = Increment(x=w206) -> (x+1=w205:i32)
            }
            frame 4 {
              (unwired) "DM "
              (unwired) "DM "
              # "Initialize deformable mirror"
              n29 = call <userlib>:"LVClass_WavefrontCorrectorSet ctor.vi"("WavefrontCorrectorSet in"=w235, "PathToWavefrontCorrectorSetupFile"=w234, "error in (no error)"=w230) -> ("WavefrontCorrectorSet out"=w242:refnum<class "WavefrontCorrectorSet.lvclass">, "error out"=w251:errorcluster)  [unwired: 11 in]
              n30 = call <userlib>:"LVClass_WavefrontCorrector ctor.vi"("WavefrontCorrector in"=w233, "PathToWavefrontCorrectorSetupFile"=w232, "error in (no error)"=w251) -> ("WavefrontCorrector out"=w239:refnum<class "WavefrontCorrector.lvclass">, "error out"=w240:errorcluster)  [unwired: 11 in]
              n31 = call <userlib>:"LVClass_WavefrontCorrector Init.vi"("WavefrontCorrector in"=w239, "set_init_state_from_config_file"=TRUE, "error in (no error)"=w240) -> ("WavefrontCorrector out"=w243:refnum<class "WavefrontCorrector.lvclass">, "error out"=w252:errorcluster)  [unwired: 11 in]
              n32 = call-poly <vilib>:"Read From Spreadsheet File.vi"("format (%.3f)"="%.8f", "file path (dialog if empty)"=w237) -> ("first row"=w254:dbl[])  [unwired: 5 in, 4 out]
              n33 = call <userlib>:"LVClass_WavefrontCorrectorSet get nb of actuators.vi"("WavefrontCorrectorSet in"=w242, "error in (no error)"=w252) -> ("WavefrontCorrectorSet out"=w228:refnum<class "WavefrontCorrectorSet.lvclass">, "ActuatorsNumber"=→"ActuatorsNumber":i32, "error out"=w253:errorcluster)  [unwired: 11 in]
              n34 = call <userlib>:"LVClass_WavefrontCorrector Get Current Preferences.vi"("WavefrontCorrector in"=w243, "error in (no error)"=w253) -> ("WavefrontCorrector out"=w248:refnum<class "WavefrontCorrector.lvclass">, "Mirror preferences.Wavefront Corrector State"=→"Initial State":T1[], "error out"=w249:errorcluster)  [unwired: 10 in, 1 out]
              n35 = case shown="True" "Initial offset" {
                tunnel: w254 -> [_ w268]
                tunnel: [w263 w267] -> w246
                tunnel: [w262 w266] -> w247
                tunnel: w248 -> [w263 w265]
                tunnel: w249 -> [w262 w264]
                frame False {
                }
                frame True {
                  n36 = call <userlib>:"LVClass_WavefrontCorrector Move to Absolute Position.vi"("WavefrontCorrector in"=w265, "Absolute Positions"=w268, "error in (no error)"=w264) -> ("WavefrontCorrector out"=w267:refnum<class "WavefrontCorrector.lvclass">, "error out"=w266:errorcluster)  [unwired: 11 in]
                }
              }
              n37 = local write "Current status"("Devices initialized") -> ()
              n38 = call <userlib>:"LVClass_WavefrontCorrector Get Current Position.vi"("WavefrontCorrector in"=w246, "error in (no error)"=w247) -> ("WavefrontCorrector out"=w231:refnum<class "WavefrontCorrector.lvclass">, "Wavefront Corrector Position"=→"Initial Positions":T14, "error out"=w229:errorcluster)  [unwired: 11 in]
              n39 = Increment(x=w227) -> (x+1=w226:i32)
            }
          }
        }
      }
    }
    n40 = local read "Exit"() -> (w57:bool)
    n41 = Or(x=w57, y="Init") -> (x .or. y?=w55:bool)
  }
  n42 = call <userlib>:"LVClass_HasoEngine ctor from file.vi"("HasoEngine in"=refnum<class "HasoEngine.lvclass"> refnum, "Configuration file path"="Haso configuration file") -> ("HasoEngine out"=w13:refnum<class "HasoEngine.lvclass">, "error out"=w14:errorcluster)  [unwired: 12 in]
  n43 = call <userlib>:"LVClass_HasoEngine Set Preferences.vi"("HasoEngine in"=w13, "Slopes_HasoEngine_Setup"=T10 {"Start sub-aperture"={"X"=16, "Y"=16}, "Pupil average"=1.0}, "error in (no error)"=w14) -> ("HasoEngine out"=w10:refnum<class "HasoEngine.lvclass">)  [unwired: 11 in, 1 out]
  n44 = while {
    shift-right: [w296] -> w46
    shift-left: w25 -> [w298]
    shift-right: [w294] -> w45
    shift-left: w38 -> [w295]
    shift-right: [w288] -> w44
    shift-left: w36 -> [w293]
    shift-right: [w287] -> w43
    shift-left: w35 -> [w292]
    shift-right: [w286] -> w42
    shift-left: w34 -> [w291]
    shift-right: [w285] -> w41
    shift-left: w33 -> [w290]
    shift-right: [w284] -> _
    shift-left: w39 -> [w289]
    shift-right: [w283] -> w40
    shift-left: w37 -> [w283]
    tunnel: w25 -> [w282]
    tunnel: w24 -> [w281]
    tunnel: w16 -> [w270]
    shift-right: [w278] -> w9
    shift-left: refnum<class "HasoSlopes.lvclass"> refnum ("HasoSlopes in") -> [w277]
    shift-right: [w276] -> w4
    shift-left: w10 -> [w279]
    shift-right: [w273] -> w5
    shift-left: refnum<class "Phase.lvclass"> refnum ("Phase in") -> [w275]
    shift-right: [w272] -> w3
    shift-left: refnum<class "Pupil.lvclass"> refnum ("Pupil in") -> [w274]
    tunnel: [w270] -> w2
    shift-right: [w269] -> w1
    shift-left: w17 -> [w271]
    stop <- w297 stop-if-true
    n45 = event shown="[6] \"Start HASO\": Mouse Up" {
      selector: _ -> [_ _ _ _ _ _ _ _ _ _ _ _ _]
      dyn-events: _ -> [_ _ _ _ _ _ _ _ _ _ _ _ _]
      timeout: 100 -> [_ _ _ _ _ _ _ _ _ _ _ _ _]
      tunnel: w298 -> [w314 w445 w448 w461 _ w508 w524 w542 w570 w661 w1140 _ w1640]
      tunnel: [w300 _ _ _ _ _ _ _ w571 w662 w1141 "Exit" TRUE ("Exit")] -> w297
      tunnel: [w301 w443 w448 w461 w479 w503 w522 w548 w569 w660 w1139 w1624 w1645] -> w296
      tunnel: w295 -> [w319 w444 w449 w462 w481 w507 w525 w549 w565 w649 w1128 w1625 w1647]
      tunnel: [w318 w442 w449 w462 w481 w504 w523 w550 w565 w649 w1128 w1623 w1646] -> w294
      tunnel: w293 -> [w322 w435 w456 w469 w483 w497 w520 w544 w581 w656 w1135 w1619 w1641]
      tunnel: w292 -> [w321 w436 w457 w470 w484 w498 w519 w545 w580 w655 w1134 w1620 w1642]
      tunnel: w291 -> [w320 w437 w458 w471 w485 w499 w518 w546 w579 w654 w1133 w1621 w1643]
      tunnel: w290 -> [w315 w438 w459 w472 w486 w500 w517 w547 w578 w653 w1132 w1622 w1644]
      tunnel: w289 -> [w311 w434 w455 w468 w482 w496 _ _ w566 w658 w1137 _ _]
      tunnel: [w317 w435 w456 w469 w483 w497 w520 w544 w581 w656 w1135 w1619 w1641] -> w288
      tunnel: [w316 w436 w457 w470 w484 w498 w519 w545 w580 w655 w1134 w1620 w1642] -> w287
      tunnel: [w313 w437 w458 w471 w485 w499 w518 w546 w579 w654 w1133 w1621 w1643] -> w286
      tunnel: [w312 w438 w459 w472 w486 w500 w517 w547 w578 w653 w1132 w1622 w1644] -> w285
      tunnel: [w311 w434 w455 w468 w482 w496 TRUE FALSE w566 w658 w1137 FALSE FALSE] -> w284
      tunnel: w282 -> [_ _ _ _ w478 _ _ _ _ _ _ _ _]
      tunnel: w281 -> [_ _ _ _ _ _ _ _ _ _ _ w1617 _]
      tunnel: w277 -> [w310 w432 w453 w466 w476 w490 w515 w540 w562 w651 w1130 w1615 w1637]
      tunnel: w279 -> [w309 w431 w452 w465 w475 w489 w514 w539 w561 w650 w1129 w1614 w1636]
      tunnel: [w308 w432 w453 w466 w476 w490 w515 w540 w562 w648 w1127 w1615 w1637] -> w278
      tunnel: [w307 w431 w452 w465 w475 w489 w514 w539 w561 w650 w1129 w1614 w1636] -> w276
      tunnel: w275 -> [w306 w433 w454 w467 w477 w491 w516 w541 w563 w652 w1131 w1616 w1638]
      tunnel: w274 -> [w305 w430 w451 w464 w474 w488 w513 w538 w560 w646 w1125 w1613 w1635]
      tunnel: [w304 w433 w454 w467 w477 w491 w516 w541 w563 w647 w1126 w1616 w1638] -> w273
      tunnel: [w303 w430 w451 w464 w474 w488 w513 w538 w560 w645 w1124 w1613 w1635] -> w272
      tunnel: w271 -> [w302 w429 w450 w463 w473 w487 w512 w537 w568 w659 w1138 w1612 w1634]
      tunnel: [w302 w429 w450 w463 w473 w487 w512 w537 w564 w657 w1136 w1612 w1634] -> w269
      event Timeout {
        n46 = event-data() -> ()  [unwired: 1 in, 2 out]
        n47 = case shown="True" w311 {
          tunnel: [w327 w348] -> w301
          tunnel: w322 -> [w332 w351]
          tunnel: [w332 w351] -> w317
          tunnel: [w328 w347] -> w316
          tunnel: w320 -> [w331 w350]
          tunnel: w315 -> [w330 w349]
          tunnel: [w331 w350] -> w313
          tunnel: [w330 w349] -> w312
          tunnel: w321 -> [w328 w347]
          tunnel: w319 -> [w329 w345]
          tunnel: [w329 w346] -> w318
          tunnel: w314 -> [w327 w344]
          tunnel: w310 -> [w325 w343]
          tunnel: w309 -> [w324 w342]
          tunnel: [w325 w341] -> w308
          tunnel: [w324 w340] -> w307
          tunnel: w306 -> [w326 w339]
          tunnel: w305 -> [w323 w338]
          tunnel: [w326 w337] -> w304
          tunnel: [w323 w336] -> w303
          frame False {
          }
          frame True {
            # "Acqure Wavefront Images"
            n48 = local read "HASO ready"() -> (w333:bool)
            n49 = And(x="Live Wavefront", y=w333) -> (x .and. y?=w335:bool)
            n50 = case shown="True" w335 {
              tunnel: w351 -> [_ w379]
              tunnel: w350 -> [_ w378]
              tunnel: w349 -> [_ w377]
              tunnel: [w352 w374] -> w348
              tunnel: w347 -> [_ w371]
              tunnel: [w357 w370] -> w346
              tunnel: w345 -> [w357 w358]
              tunnel: w344 -> [w352 w359]
              tunnel: w343 -> [w355 w369]
              tunnel: w342 -> [w354 w368]
              tunnel: [w355 w367] -> w341
              tunnel: [w354 w366] -> w340
              tunnel: w339 -> [w356 w365]
              tunnel: w338 -> [w353 w364]
              tunnel: [w356 w363] -> w337
              tunnel: [w353 w362] -> w336
              frame False {
              }
              frame True {
                n51 = property on="nb_images (set)" class="DigNum (strict)"() -> ("Value"=w380:u32)  [unwired: 2 in, 2 out]
                n52 = case shown="1" w380 {
                  tunnel: [w426 w428] -> w381
                  tunnel: w371 -> [w425 _]
                  tunnel: w379 -> [w426 _]
                  tunnel: [w425 w427] -> w376
                  tunnel: w378 -> [_ w428]
                  tunnel: w377 -> [_ w427]
                  frame 2, Default {
                  }
                  frame 1 {
                  }
                }
                n53 = call <userlib>:"LVClass_Camera get image.vi"("Camera in"=w358, "Image"=w381, "Image RAW"=w376, "remove_background"=FALSE, "error in (no error)"=w359) -> ("Camera out"=w370:refnum<class "Camera.lvclass">, "Image (dup)"=w375:refnum<class "Image.lvclass">, "error out"=w372:errorcluster)  [unwired: 7 in, 1 out]
                n54 = case shown="No Error" w372 {
                  selector: w372 -> [w422 w423]
                  tunnel: w375 -> [w419 w424]
                  tunnel: [w417 w424] -> w361
                  tunnel: [w416 w423] -> w360
                  frame No Error {
                    # "get image"
                    n55 = call <userlib>:"LVClass_Image get image data.vi"("Image in"=w419, "error in (no error)"=w422) -> ("Image out"=w421:refnum<class "Image.lvclass">, "Image data out"=w415:u32[][], "error out"=w420:errorcluster)  [unwired: 11 in]
                    n56 = call <userlib>:"LVClass_Image get image information.vi"("Image in"=w421, "error in (no error)"=w420) -> ("Image out"=w417:refnum<class "Image.lvclass">, "Acquisition information"=→"Acquisition information":T5, "error out"=w416:errorcluster)  [unwired: 11 in]
                    n57 = local write "HASO intensity"(w415) -> ()
                  }
                  frame Error {
                  }
                }
                n58 = case shown="No Error" w360 {
                  selector: w360 -> [w402 w414]
                  tunnel: [w408 w414] -> w374
                  tunnel: w361 -> [w401 _]
                  tunnel: [w406 w410] -> w362
                  tunnel: [w405 w413] -> w363
                  tunnel: w369 -> [w398 w412]
                  tunnel: w368 -> [w397 w411]
                  tunnel: [w386 w412] -> w367
                  tunnel: [w396 w411] -> w366
                  tunnel: w365 -> [w394 w413]
                  tunnel: w364 -> [w392 w410]
                  frame No Error {
                    # "phaseout"
                    n59 = call "image2slopes.vi"("error in (no error)"=w402, "Image in"=w401, "HasoEngine in"=w397, "HasoSlopes in"=w398) -> ("error out"=w395:errorcluster, "HasoEngine out"=w396:refnum<class "HasoEngine.lvclass">, "HasoSlopes out"=w388:refnum<class "HasoSlopes.lvclass">)  [unwired: 4 in, 1 out]
                    n60 = local read "Filter"() -> (w391:u8[])
                    n61 = call "slopes2phase.vi"("TypePhase"=WavefrontReconstructionMode."Modal_Zernike", "Number of coefficients"=u8 32, "error in (no error)"=w395, "Filter"=w391, "HasoSlopes in"=w388, "Phase in"=w394) -> ("error out"=w385:errorcluster, "HasoSlopes out"=w387:refnum<class "HasoSlopes.lvclass">, "Phase out"=w393:refnum<class "Phase.lvclass">)  [unwired: 3 in]
                    n62 = local read "idxType"() -> (w382:enum16{"Wyant", "ANSI"})
                    n63 = call "slopes2zern.vi"("HasoSlopes in"=w387, "error in (no error)"=w385, "idxType"=w382) -> ("HasoSlopes out"=w386:refnum<class "HasoSlopes.lvclass">, "Zernike Coefficients"=w383:dbl[], "error out"=w384:errorcluster)  [unwired: 3 in, 2 out]
                    n64 = call <userlib>:"LVClass_Pupil ctor from HasoSlopes.vi"("Pupil in"=w392, "HasoSlopes.lvclass"=w388, "error in (no error)"=w384) -> ("Pupil out"=w403:refnum<class "Pupil.lvclass">, "error out"=w404:errorcluster)  [unwired: 11 in]
                    n65 = call <userlib>:"LVClasse_Phase GetStatisticDatas.vi"("Phase in"=w393, "error in (no error)"=w404) -> ("Phase out"=w409:refnum<class "Phase.lvclass">, "StatisticsData"=w389:T2, "error out"=w407:errorcluster)  [unwired: 11 in]
                    n66 = local write "Phase statistics"(w389) -> ()
                    n67 = call <userlib>:"LVClasse_Phase Get Data.vi"("Phase in"=w409, "Pupil"=w403, "error in (no error)"=w407) -> ("Phase out"=w405:refnum<class "Phase.lvclass">, "data"=w390:sgl[][], "Pupil (dup)"=w406:refnum<class "Pupil.lvclass">, "error out"=w408:errorcluster)  [unwired: 9 in]
                    n68 = local write "Zernike Measured"(w383) -> ()
                    n69 = local write "Phase values"(w390) -> ()
                  }
                  frame Error {
                  }
                }
              }
            }
          }
        }
        "Current error" <- w301
        n70 = Unbundle By Name(w301) -> ("status"=w300:bool)
      }
      event "nb_images (set)": Value Change {
        # "SET IMAGE NUMBER"
        n71 = event-data() -> ("NewVal"=w446:u32)  [unwired: 1 in]
        n72 = call <userlib>:"LVClass_Camera set nbImagesToSum.vi"("Camera in"=w444, "nb_image"=w446, "error in (no error)"=w445) -> ("Camera out"=w441:refnum<class "Camera.lvclass">, "error out"=w440:errorcluster)  [unwired: 11 in]
        n73 = call <userlib>:"LVClass_Camera get nbImagesToSum.vi"("Camera in"=w441, "error in (no error)"=w440) -> ("Camera out"=w442:refnum<class "Camera.lvclass">, "nb_image"=→"nb_images (get)":u32, "error out"=w443:errorcluster)  [unwired: 11 in]
      }
      event "Coef Min": Value Change {
        # "Set coeff display scale: min"
        n74 = event-data() -> ()  [unwired: 1 in, 1 out]
        n75 = local read "Coef Min"() -> (w447:dbl)
        n76 = property on="Zernike Measured" class="WFGraph (strict)"("YScale.Minimum"=w447) -> ()  [unwired: 2 in, 2 out]
      }
      event "Coef Max": Value Change {
        # "Set coeff display scale: min"
        n77 = event-data() -> ()  [unwired: 1 in, 1 out]
        n78 = local read "Coef Max"() -> (w460:dbl)
        n79 = property on="Zernike Measured" class="WFGraph (strict)"("YScale.Maximum"=w460) -> ()  [unwired: 2 in, 2 out]
      }
      event "Reset error": Mouse Up {
        n80 = event-data() -> ()  [unwired: 1 in, 8 out]
        n81 = Select(t=w478, s=w478, f=errorcluster {"status"=FALSE, "code"=0, "source"=""} ("error out")) -> (s? t:f=w479:errorcluster)
      }
      event "exposure_duration_s (set)": Value Change {
        # "CHANGE EXPOSURE DURATION"
        n82 = event-data() -> ()  [unwired: 1 in, 1 out]
        n83 = Multiply(x=1000000.0, y="exposure_duration_s (set)") -> (x*y=w494:dbl)
        n84 = To Unsigned Long Integer(number=w494) -> (unsigned 32bit integer=w493:u32)
        n85 = call <userlib>:"LVClass_Camera set Parameter Int.vi"("Camera in"=w507, "parameter_name"="exposure_duration_us", "value"=w493, "error in (no error)"=w508) -> ("Camera out"=w506:refnum<class "Camera.lvclass">, "error out"=w505:errorcluster)  [unwired: 10 in]
        n86 = call <userlib>:"LVClass_Camera get Parameter Int.vi"("Camera in"=w506, "parameter_name"="exposure_duration_us", "error in (no error)"=w505) -> ("Camera out"=w504:refnum<class "Camera.lvclass">, "value"=→"exposure_duration_us (get)":i32, "error out"=w503:errorcluster)  [unwired: 10 in]
      }
      event "Start HASO": Mouse Up {
        # "Does NOT work when exp time > 0.1ms"
        # "Start acquisition in SYNCRHONOUS mode\n\nSet mode as: new_image"
        n87 = event-data() -> ()  [unwired: 1 in, 8 out]
        n88 = flat-sequence {
          tunnel: w525 -> [w531]
          tunnel: w524 -> [w530]
          tunnel: [w529] -> w511
          tunnel: [w528] -> w510
          tunnel: [w533] -> w522
          tunnel: [w534] -> w523
          tunnel: w511 -> [w534]
          tunnel: w510 -> [w533]
          frame #0 {
            n89 = call <userlib>:"LVClass_Camera start acquisition.vi"("Camera in"=w531, "synchronisation_mode"=enum16{"synchronous", "asynchronous"}."synchronous", "acquisition_mode"=enum16{"last_image", "new_image"}."new_image", "error in (no error)"=w530) -> ("Camera out"=w529:refnum<class "Camera.lvclass">, "error out"=w528:errorcluster)  [unwired: 10 in]
          }
          frame #1 {
            n90 = local write "HASO ready"(TRUE) -> ()
          }
        }
      }
      event "Stop HASO": Mouse Up {
        n91 = event-data() -> ()  [unwired: 1 in, 8 out]
        n92 = flat-sequence {
          tunnel: w549 -> [w553]
          tunnel: w542 -> [w551]
          tunnel: [w554] -> w536
          tunnel: [w552] -> w535
          tunnel: [w556] -> w548
          tunnel: [w557] -> w550
          tunnel: w536 -> [w557]
          tunnel: w535 -> [w556]
          frame #0 {
            n93 = call <userlib>:"LVClass_Camera stop acquisition.vi"("Camera in"=w553, "error in (no error)"=w551) -> ("Camera out"=w554:refnum<class "Camera.lvclass">, "error out"=w552:errorcluster)  [unwired: 12 in]
          }
          frame #1 {
            n94 = local write "HASO ready"(FALSE) -> ()
          }
        }
      }
      event "Update DM": Mouse Up {
        n95 = event-data() -> ()  [unwired: 1 in, 8 out]
        n96 = local read "Initial offset"() -> (w567:bool)
        n97 = case shown="True" w567 {
          tunnel: [w582 w587] -> w572
          frame False {
            n98 = Initialize Array(0.0, 52) -> (w582:dbl[])
          }
          frame True {
            n99 = local read "Offset command file"() -> (w586:path)
            n100 = call-poly <vilib>:"Read From Spreadsheet File.vi"("format (%.3f)"="%.8f", "file path (dialog if empty)"=w586) -> ("first row"=w587:dbl[])  [unwired: 5 in, 4 out]
          }
        }
        n101 = local read "Additional Command"() -> (w577:bool)
        n102 = case shown="True" w577 {
          tunnel: [w589 w595] -> w573
          tunnel: [w588 w594] -> w574
          tunnel: w570 -> [w588 w593]
          frame False {
            n103 = Initialize Array(0.0, 52) -> (w589:dbl[])
          }
          frame True {
            n104 = local read "Input type"() -> (w592:T4)
            n105 = case shown="\"Zero Input\"" w592 {
              tunnel: w593 -> [w596 w601 w615 w624]
              tunnel: [w597 w602 w613 w626] -> w595
              tunnel: [w596 w601 w612 w623] -> w594
              frame "Zero Input" {
                n106 = Initialize Array(0.0, 52) -> (w597:dbl[])
              }
              frame "Command File" {
                n107 = local read "Additional file"() -> (w600:path)
                n108 = call-poly <vilib>:"Read From Spreadsheet File.vi"("format (%.3f)"="%.8f", "file path (dialog if empty)"=w600) -> ("first row"=w602:dbl[])  [unwired: 5 in, 4 out]
              }
              frame "Zernike Coef", Default {
                n109 = local read "Zern index in"() -> (w604:i32[])
                n110 = local read "Zern coef in"() -> (w605:sgl[])
                n111 = local read "idxType"() -> (w611:enum16{"Wyant", "ANSI"})
                n112 = local read "Initial haso file"() -> (w609:path)
                n113 = local read "Haso configuration file"() -> (w610:path)
                n114 = local read "interaction matrix file"() -> (w608:path)
                n115 = call "zern2command.vi"("Haso configuration file"=w610, "idxType"=w611, "interaction matrix file"=w608, "error in (no error)"=w615, "Zern coef in"=w605, "Zern index in"=w604, "Initial haso file"=w609) -> ("error out"=w614:errorcluster, "Offset Positions"=w613:sgl[], "Zern pupil out"=w616:refnum<class "Pupil.lvclass">, "ModalCoef out"=w617:refnum<class "ModalCoef.lvclass">)  [unwired: 1 in]
                n116 = call <userlib>:"LVClass_ModalCoef GetData.vi"("ModalCoef in"=w617, "Pupil.lvclass"=w616, "error in (no error)"=w614) -> ("ModalCoef out"=w621:refnum<class "ModalCoef.lvclass">, "coef"=w607:sgl[], "index"=w606:u32[], "Pupil.lvclass (dup)"=w620:refnum<class "Pupil.lvclass">, "error out"=w619:errorcluster)  [unwired: 8 in]
                n117 = local write "Zern index out"(w606) -> ()
                n118 = call <userlib>:"LVClass_Pupil dtor.vi"("Pupil in"=w620, "error in (no error)"=w619) -> ("error out"=w618:errorcluster)  [unwired: 12 in, 1 out]
                n119 = local write "Zern coef out"(w607) -> ()
                n120 = call <userlib>:"LVClass_ModalCoef dtor.vi"("ModalCoef in"=w621, "error in (no error)"=w618) -> ("error out"=w612:errorcluster)  [unwired: 12 in, 1 out]
              }
              frame "Zernike File" {
                w629 = 1
                n121 = local read "interaction matrix file"() -> (w633:path)
                n122 = local read "Initial haso file"() -> (w631:path)
                n123 = local read "Haso configuration file"() -> (w632:path)
                n124 = local read "Additional file"() -> (w642:path)
                n125 = call-poly <vilib>:"Ramp Pattern.vi"("start"=w629, "end"=32, "delta"=w629) -> ("Ramp Pattern"=w630:dbl[])  [unwired: 6 in, 2 out]
                n126 = To Long Integer(number=w630) -> (32bit integer=w627:i32[])
                n127 = local read "idxType"() -> (w622:enum16{"Wyant", "ANSI"})
                n128 = call-poly <vilib>:"Read From Spreadsheet File.vi"("format (%.3f)"="%.8f", "file path (dialog if empty)"=w642) -> ("first row"=w634:dbl[])  [unwired: 5 in, 4 out]
                n129 = call "zern2command.vi"("Haso configuration file"=w632, "idxType"=w622, "interaction matrix file"=w633, "Zern coef in"=w634, "Zern index in"=w627, "Initial haso file"=w631) -> ("error out"=w635:errorcluster, "Offset Positions"=w626:sgl[], "Zern pupil out"=w636:refnum<class "Pupil.lvclass">, "ModalCoef out"=w637:refnum<class "ModalCoef.lvclass">)  [unwired: 2 in]
                n130 = call <userlib>:"LVClass_ModalCoef GetData.vi"("ModalCoef in"=w637, "Pupil.lvclass"=w636, "error in (no error)"=w635) -> ("ModalCoef out"=w641:refnum<class "ModalCoef.lvclass">, "Pupil.lvclass (dup)"=w640:refnum<class "Pupil.lvclass">, "error out"=w639:errorcluster)  [unwired: 8 in, 2 out]
                n131 = call <userlib>:"LVClass_Pupil dtor.vi"("Pupil in"=w640, "error in (no error)"=w639) -> ("error out"=w638:errorcluster)  [unwired: 12 in, 1 out]
                n132 = call <userlib>:"LVClass_ModalCoef dtor.vi"("ModalCoef in"=w641, "error in (no error)"=w638) -> ("error out"=w625:errorcluster)  [unwired: 12 in, 1 out]
                n133 = Merge Errors(w625, w624) -> (w623:errorcluster)
              }
            }
          }
        }
        n134 = local write "Initial Positions"(w572) -> ()
        n135 = Add(x=w573, y=w572) -> (x+y=w558:dbl[])
        n136 = call <userlib>:"LVClass_WavefrontCorrector Move to Absolute Position.vi"("WavefrontCorrector in"=w568, "Absolute Positions"=w558, "error in (no error)"=w574) -> ("WavefrontCorrector out"=w575:refnum<class "WavefrontCorrector.lvclass">, "error out"=w576:errorcluster)  [unwired: 11 in]
        n137 = call <userlib>:"LVClass_WavefrontCorrector Get Current Position.vi"("WavefrontCorrector in"=w575, "error in (no error)"=w576) -> ("WavefrontCorrector out"=w564:refnum<class "WavefrontCorrector.lvclass">, "Wavefront Corrector Position"=w559:T14, "error out"=w569:errorcluster)  [unwired: 11 in]
        n138 = local write "Final Positions"(w558) -> ()
        n139 = local write "DM Actuator Values"(w559) -> ()
        n140 = Unbundle By Name(w569) -> ("status"=w571:bool)
      }
      event "Record Response": Mouse Up {
        n141 = event-data() -> ()  [unwired: 1 in, 8 out]
        n142 = local read "Net Rp"() -> (w644:bool)
        n143 = stacked-sequence {
          seq-local: [_ _ _ w960 _] -> [_ _ _ _ w985]
          seq-local: [_ _ w849 _ _] -> [_ _ _ w959 _]
          seq-local: [_ w687 _ _ _] -> [_ _ w850 _ _]
          seq-local: [_ _ w848 _ _] -> [_ _ _ _ w981]
          tunnel: [_ _ _ _ w984] -> w662
          tunnel: w661 -> [_ w700 _ _ _]
          tunnel: [_ _ _ _ w983] -> w660
          tunnel: w659 -> [_ w699 _ w961 _]
          tunnel: [_ w697 _ _ _] -> w657
          tunnel: w656 -> [_ _ w862 _ w993]
          tunnel: w655 -> [_ _ w861 _ w992]
          tunnel: w654 -> [_ _ w860 _ w991]
          tunnel: w653 -> [_ _ w859 _ w990]
          tunnel: w652 -> [_ _ w858 _ w989]
          tunnel: w651 -> [_ _ w857 _ _]
          tunnel: w650 -> [_ _ w856 _ w988]
          tunnel: w646 -> [_ _ w855 _ w987]
          tunnel: w649 -> [_ _ w854 _ w986]
          tunnel: [_ _ _ _ w980] -> w648
          tunnel: [_ _ w852 _ _] -> w647
          tunnel: [_ _ w851 _ _] -> w645
          tunnel: w644 -> [_ _ _ w958 w982]
          frame #0 {
            # "Create output folder path"
            n144 = Get Date/Time In Seconds() -> (seconds since 1Jan1904=w674:timestamp)
            n145 = local read "Folder Name"() -> (w666:string)
            n146 = Format Date/Time String(time format string (%c)="%Y%m%d", seconds (now)=w674) -> (date/time string=w673:string)  [unwired: 1 in]
            n147 = local read "Main Path"() -> (w667:path)
            n148 = local read "Subfolder"() -> (w665:string)
            n149 = Concatenate Strings(w673, "_", w666) -> (w672:string)
            n150 = Build Path(base path=w667, name or relative path=w672) -> (appended path=w670:path)
            n151 = call <vilib>:"Check if File or Folder Exists.vi"("path"=w670) -> ("file or folder exists?"=w676:bool)  [unwired: 8 in, 2 out]
            n152 = local write "Current status"("Check single response") -> ()
            n153 = Build Path(base path=w670, name or relative path=w665) -> (appended path=w664:path)
            n154 = case shown="False" w676 {
              tunnel: w670 -> [w686 _]
              frame False {
                n155 = Create Folder(path (use dialog)=w686) -> ()  [unwired: 2 in, 3 out]
              }
              frame True {
              }
            }
            n156 = call <vilib>:"Check if File or Folder Exists.vi"("path"=w664) -> ("error out"=w671:errorcluster, "file or folder exists?"=w675:bool)  [unwired: 8 in, 1 out]
            n157 = case shown="True" w675 {
              tunnel: w664 -> [w679 w684]
              tunnel: w671 -> [w678 w685]
              tunnel: [w677 w680] -> _
              frame False {
                n158 = Create Folder(path (use dialog)=w679, error in=w678) -> (error out=w677:errorcluster)  [unwired: 1 in, 2 out]
              }
              frame True {
                n159 = Delete(path (use dialog)=w684, entire hierarchy (F)=TRUE, error in=w685) -> (deleted path=w682:path, error out=w681:errorcluster)  [unwired: 2 in, 1 out]
                n160 = Create Folder(path (use dialog)=w682, error in=w681) -> (error out=w680:errorcluster)  [unwired: 1 in, 2 out]
              }
            }
            n161 = local write "Output path"(w664) -> ()
          }
          frame #1 {
            # "Delay for DM response"
            # "Apply command to DM"
            n162 = local read "Initial offset"() -> (w698:bool)
            n163 = case shown="True" w698 {
              tunnel: [w786 w791] -> w689
              frame False {
                n164 = Initialize Array(0.0, 52) -> (w786:dbl[])
              }
              frame True {
                n165 = local read "Offset command file"() -> (w790:path)
                n166 = call-poly <vilib>:"Read From Spreadsheet File.vi"("format (%.3f)"="%.8f", "file path (dialog if empty)"=w790) -> ("first row"=w791:dbl[])  [unwired: 5 in, 4 out]
              }
            }
            n167 = local read "Additional Command"() -> (w704:bool)
            n168 = case shown="True" w704 {
              tunnel: [w793 w799] -> w690
              tunnel: [w792 w798] -> w701
              tunnel: w700 -> [w792 w797]
              frame False {
                n169 = Initialize Array(0.0, 52) -> (w793:dbl[])
              }
              frame True {
                n170 = local read "Input type"() -> (w796:T4)
                n171 = case shown="\"Zernike Coef\", Default" w796 {
                  tunnel: w797 -> [w800 w805 w819 w828]
                  tunnel: [w801 w806 w817 w830] -> w799
                  tunnel: [w800 w805 w816 w827] -> w798
                  frame "Zero Input" {
                    n172 = Initialize Array(0.0, 52) -> (w801:dbl[])
                  }
                  frame "Command File" {
                    n173 = local read "Additional file"() -> (w804:path)
                    n174 = call-poly <vilib>:"Read From Spreadsheet File.vi"("format (%.3f)"="%.8f", "file path (dialog if empty)"=w804) -> ("first row"=w806:dbl[])  [unwired: 5 in, 4 out]
                  }
                  frame "Zernike Coef", Default {
                    n175 = local read "Zern index in"() -> (w808:i32[])
                    n176 = local read "Zern coef in"() -> (w809:sgl[])
                    n177 = local read "idxType"() -> (w815:enum16{"Wyant", "ANSI"})
                    n178 = local read "Initial haso file"() -> (w813:path)
                    n179 = local read "Haso configuration file"() -> (w814:path)
                    n180 = local read "interaction matrix file"() -> (w812:path)
                    n181 = call "zern2command.vi"("Haso configuration file"=w814, "idxType"=w815, "interaction matrix file"=w812, "error in (no error)"=w819, "Zern coef in"=w809, "Zern index in"=w808, "Initial haso file"=w813) -> ("error out"=w818:errorcluster, "Offset Positions"=w817:sgl[], "Zern pupil out"=w820:refnum<class "Pupil.lvclass">, "ModalCoef out"=w821:refnum<class "ModalCoef.lvclass">)  [unwired: 1 in]
                    n182 = call <userlib>:"LVClass_ModalCoef GetData.vi"("ModalCoef in"=w821, "Pupil.lvclass"=w820, "error in (no error)"=w818) -> ("ModalCoef out"=w825:refnum<class "ModalCoef.lvclass">, "coef"=w811:sgl[], "index"=w810:u32[], "Pupil.lvclass (dup)"=w824:refnum<class "Pupil.lvclass">, "error out"=w823:errorcluster)  [unwired: 8 in]
                    n183 = local write "Zern index out"(w810) -> ()
                    n184 = call <userlib>:"LVClass_Pupil dtor.vi"("Pupil in"=w824, "error in (no error)"=w823) -> ("error out"=w822:errorcluster)  [unwired: 12 in, 1 out]
                    n185 = local write "Zern coef out"(w811) -> ()
                    n186 = call <userlib>:"LVClass_ModalCoef dtor.vi"("ModalCoef in"=w825, "error in (no error)"=w822) -> ("error out"=w816:errorcluster)  [unwired: 12 in, 1 out]
                  }
                  frame "Zernike File" {
                    w833 = 1
                    n187 = local read "interaction matrix file"() -> (w837:path)
                    n188 = local read "Initial haso file"() -> (w835:path)
                    n189 = local read "Haso configuration file"() -> (w836:path)
                    n190 = local read "Additional file"() -> (w846:path)
                    n191 = call-poly <vilib>:"Ramp Pattern.vi"("start"=w833, "end"=32, "delta"=w833) -> ("Ramp Pattern"=w834:dbl[])  [unwired: 6 in, 2 out]
                    n192 = To Long Integer(number=w834) -> (32bit integer=w831:i32[])
                    n193 = local read "idxType"() -> (w826:enum16{"Wyant", "ANSI"})
                    n194 = call-poly <vilib>:"Read From Spreadsheet File.vi"("format (%.3f)"="%.8f", "file path (dialog if empty)"=w846) -> ("first row"=w838:dbl[])  [unwired: 5 in, 4 out]
                    n195 = call "zern2command.vi"("Haso configuration file"=w836, "idxType"=w826, "interaction matrix file"=w837, "Zern coef in"=w838, "Zern index in"=w831, "Initial haso file"=w835) -> ("error out"=w839:errorcluster, "Offset Positions"=w830:sgl[], "Zern pupil out"=w840:refnum<class "Pupil.lvclass">, "ModalCoef out"=w841:refnum<class "ModalCoef.lvclass">)  [unwired: 2 in]
                    n196 = call <userlib>:"LVClass_ModalCoef GetData.vi"("ModalCoef in"=w841, "Pupil.lvclass"=w840, "error in (no error)"=w839) -> ("ModalCoef out"=w845:refnum<class "ModalCoef.lvclass">, "Pupil.lvclass (dup)"=w844:refnum<class "Pupil.lvclass">, "error out"=w843:errorcluster)  [unwired: 8 in, 2 out]
                    n197 = call <userlib>:"LVClass_Pupil dtor.vi"("Pupil in"=w844, "error in (no error)"=w843) -> ("error out"=w842:errorcluster)  [unwired: 12 in, 1 out]
                    n198 = call <userlib>:"LVClass_ModalCoef dtor.vi"("ModalCoef in"=w845, "error in (no error)"=w842) -> ("error out"=w829:errorcluster)  [unwired: 12 in, 1 out]
                    n199 = Merge Errors(w829, w828) -> (w827:errorcluster)
                  }
                }
              }
            }
            n200 = local read "File Base Name"() -> (w691:string)
            n201 = local read "Output path"() -> (w695:path)
            n202 = local read "Input type"() -> (w692:T4)
            n203 = local read "Save File"() -> (w696:bool)
            n204 = local write "Initial Positions"(w689) -> ()
            n205 = Add(x=w690, y=w689) -> (x+y=w693:dbl[])
            n206 = call <userlib>:"LVClass_WavefrontCorrector Move to Absolute Position.vi"("WavefrontCorrector in"=w699, "Absolute Positions"=w693, "error in (no error)"=w701) -> ("WavefrontCorrector out"=w702:refnum<class "WavefrontCorrector.lvclass">, "error out"=w703:errorcluster)  [unwired: 11 in]
            n207 = call <userlib>:"LVClass_WavefrontCorrector Get Current Position.vi"("WavefrontCorrector in"=w702, "error in (no error)"=w703) -> ("WavefrontCorrector out"=w697:refnum<class "WavefrontCorrector.lvclass">, "Wavefront Corrector Position"=w694:T14, "error out"=w688:errorcluster)  [unwired: 11 in]
            n208 = case shown="True" w696 {
              tunnel: w695 -> [_ w713]
              tunnel: w691 -> [_ w712]
              tunnel: w689 -> [_ w711]
              tunnel: w690 -> [_ w710]
              tunnel: w693 -> [_ w709]
              tunnel: w692 -> [_ w708]
              tunnel: w694 -> [_ w707]
              frame False {
              }
              frame True {
                n209 = stacked-sequence {
                  tunnel: w713 -> [w718 w727 w736 w745 w752 w764 w776]
                  tunnel: w712 -> [w716 w725 w734 w743 w751 w763 w775]
                  tunnel: w711 -> [w714 _ _ _ _ _ _]
                  tunnel: w710 -> [_ w723 _ _ _ _ _]
                  tunnel: w709 -> [_ _ w732 _ _ _ _]
                  tunnel: w708 -> [_ _ _ _ w750 w762 w774]
                  tunnel: w707 -> [_ _ _ w741 _ _ _]
                  frame #0 {
                    n210 = Concatenate Strings(w716, "_cmdOffset", ".dat") -> (w719:string)
                    n211 = Build Path(base path=w718, name or relative path=w719) -> (appended path=w720:path)
                    n212 = Array To Spreadsheet String(array=w714, 3:"%f") -> (spreadsheet string=w721:string)  [unwired: 1 in]
                    n213 = Write to Text File(file (use dialog)=w720, text=w721) -> ()  [unwired: 2 in, 3 out]
                  }
                  frame #1 {
                    n214 = Concatenate Strings(w725, "_cmdAdd", ".dat") -> (w728:string)
                    n215 = Build Path(base path=w727, name or relative path=w728) -> (appended path=w729:path)
                    n216 = Array To Spreadsheet String(array=w723, 3:"%f") -> (spreadsheet string=w730:string)  [unwired: 1 in]
                    n217 = Write to Text File(file (use dialog)=w729, text=w730) -> ()  [unwired: 2 in, 3 out]
                  }
                  frame #2 {
                    n218 = Concatenate Strings(w734, "_cmdFinal", ".dat") -> (w737:string)
                    n219 = Build Path(base path=w736, name or relative path=w737) -> (appended path=w738:path)
                    n220 = Array To Spreadsheet String(array=w732, 3:"%f") -> (spreadsheet string=w739:string)  [unwired: 1 in]
                    n221 = Write to Text File(file (use dialog)=w738, text=w739) -> ()  [unwired: 2 in, 3 out]
                  }
                  frame #3 {
                    n222 = Concatenate Strings(w743, "_cmdFinalMirror", ".dat") -> (w746:string)
                    n223 = Build Path(base path=w745, name or relative path=w746) -> (appended path=w747:path)
                    n224 = Array To Spreadsheet String(array=w741, 3:"%f") -> (spreadsheet string=w748:string)  [unwired: 1 in]
                    n225 = Write to Text File(file (use dialog)=w747, text=w748) -> ()  [unwired: 2 in, 3 out]
                  }
                  frame #4 {
                    n226 = case shown="\"Zernike Coef\", Default" w750 {
                      tunnel: w752 -> [_ w757]
                      tunnel: w751 -> [_ w755]
                      frame "Zero Input" {
                      }
                      frame "Zernike Coef", Default {
                        n227 = local read "Zern coef in"() -> (w753:sgl[])
                        n228 = Concatenate Strings(w755, "_zernCoef", ".txt") -> (w758:string)
                        n229 = Build Path(base path=w757, name or relative path=w758) -> (appended path=w759:path)
                        n230 = Array To Spreadsheet String(array=w753, 3:"%f") -> (spreadsheet string=w760:string)  [unwired: 1 in]
                        n231 = Write to Text File(file (use dialog)=w759, text=w760) -> ()  [unwired: 2 in, 3 out]
                      }
                    }
                  }
                  frame #5 {
                    n232 = case shown="\"Zernike Coef\", Default" w762 {
                      tunnel: w764 -> [_ w769]
                      tunnel: w763 -> [_ w767]
                      frame "Zero Input" {
                      }
                      frame "Zernike Coef", Default {
                        n233 = local read "Zern index in"() -> (w765:i32[])
                        n234 = Concatenate Strings(w767, "_zernIdx", ".txt") -> (w770:string)
                        n235 = Build Path(base path=w769, name or relative path=w770) -> (appended path=w771:path)
                        n236 = Array To Spreadsheet String(array=w765, 3:"%d") -> (spreadsheet string=w772:string)  [unwired: 1 in]
                        n237 = Write to Text File(file (use dialog)=w771, text=w772) -> ()  [unwired: 2 in, 3 out]
                      }
                    }
                  }
                  frame #6 {
                    n238 = case shown="\"Zernike Coef\", Default" w774 {
                      tunnel: w776 -> [_ w781]
                      tunnel: w775 -> [_ w779]
                      frame "Zero Input" {
                      }
                      frame "Zernike Coef", Default {
                        n239 = Concatenate Strings(w779, "_zernCoefWyant", ".txt") -> (w782:string)
                        n240 = local read "Zern coef out"() -> (w777:sgl[])
                        n241 = Build Path(base path=w781, name or relative path=w782) -> (appended path=w783:path)
                        n242 = Array To Spreadsheet String(array=w777, 3:"%f") -> (spreadsheet string=w784:string)  [unwired: 1 in]
                        n243 = Write to Text File(file (use dialog)=w783, text=w784) -> ()  [unwired: 2 in, 3 out]
                      }
                    }
                  }
                }
              }
            }
            n244 = local write "Final Positions"(w693) -> ()
            n245 = local write "DM Actuator Values"(w694) -> ()
            n246 = flat-sequence {
              tunnel: [w705] -> w687
              tunnel: w688 -> [w705]
              frame #0 {
                n247 = Wait (ms)(milliseconds to wait=u32 50) -> ()  [unwired: 1 out]
              }
            }
          }
          frame #2 {
            n248 = local read "HASO ready"() -> (w853:bool)
            n249 = case shown="True" w853 {
              tunnel: w862 -> [_ w888]
              tunnel: w860 -> [_ w887]
              tunnel: w859 -> [_ w886]
              tunnel: [w863 w883] -> w849
              tunnel: w861 -> [_ w881]
              tunnel: w854 -> [_ w868]
              tunnel: w850 -> [w863 w869]
              tunnel: w857 -> [w866 w880]
              tunnel: w856 -> [w865 w879]
              tunnel: [w866 w878] -> w848
              tunnel: [w865 w877] -> _
              tunnel: w858 -> [w867 w876]
              tunnel: w855 -> [w864 w875]
              tunnel: [w867 w874] -> w852
              tunnel: [w864 w873] -> w851
              frame False {
              }
              frame True {
                n250 = property on="nb_images (set)" class="DigNum (strict)"() -> ("Value"=w889:u32)  [unwired: 2 in, 2 out]
                n251 = case shown="2, Default" w889 {
                  tunnel: [w955 w957] -> w890
                  tunnel: w881 -> [w954 _]
                  tunnel: w888 -> [w955 _]
                  tunnel: [w954 w956] -> w885
                  tunnel: w887 -> [_ w957]
                  tunnel: w886 -> [_ w956]
                  frame 2, Default {
                  }
                  frame 1 {
                  }
                }
                n252 = call <userlib>:"LVClass_Camera get image.vi"("Camera in"=w868, "Image"=w890, "Image RAW"=w885, "remove_background"=FALSE, "error in (no error)"=w869) -> ("Image (dup)"=w884:refnum<class "Image.lvclass">, "error out"=w882:errorcluster)  [unwired: 7 in, 2 out]
                n253 = case shown="No Error" w882 {
                  selector: w882 -> [w951 w952]
                  tunnel: w884 -> [w950 w953]
                  tunnel: [w947 w953] -> w872
                  tunnel: [w948 w952] -> w871
                  frame No Error {
                    # "get image"
                    n254 = call <userlib>:"LVClass_Image get image data.vi"("Image in"=w950, "error in (no error)"=w951) -> ("Image out"=w947:refnum<class "Image.lvclass">, "Image data out"=w949:u32[][], "error out"=w948:errorcluster)  [unwired: 11 in]
                    n255 = local write "HASO intensity"(w949) -> ()
                  }
                  frame Error {
                  }
                }
                n256 = case shown="No Error" w871 {
                  selector: w871 -> [w914 w946]
                  tunnel: [w920 w946] -> w883
                  tunnel: w872 -> [w913 _]
                  tunnel: [w918 w942] -> w873
                  tunnel: [w917 w945] -> w874
                  tunnel: w880 -> [w910 w944]
                  tunnel: w879 -> [w909 w943]
                  tunnel: [w897 w944] -> w878
                  tunnel: [w908 w943] -> w877
                  tunnel: w876 -> [w906 w945]
                  tunnel: w875 -> [w904 w942]
                  frame No Error {
                    # "phaseout"
                    n257 = local read "File Base Name"() -> (w895:string)
                    n258 = local read "Save File"() -> (w896:bool)
                    n259 = local read "Output path"() -> (w894:path)
                    n260 = call "image2slopes.vi"("error in (no error)"=w914, "Image in"=w913, "HasoEngine in"=w909, "HasoSlopes in"=w910) -> ("error out"=w907:errorcluster, "HasoEngine out"=w908:refnum<class "HasoEngine.lvclass">, "HasoSlopes out"=w891:refnum<class "HasoSlopes.lvclass">)  [unwired: 4 in, 1 out]
                    n261 = local read "Filter"() -> (w903:u8[])
                    n262 = call "slopes2phase.vi"("TypePhase"=WavefrontReconstructionMode."Modal_Zernike", "Number of coefficients"=u8 32, "error in (no error)"=w907, "Filter"=w903, "HasoSlopes in"=w891, "Phase in"=w906) -> ("error out"=w899:errorcluster, "HasoSlopes out"=w900:refnum<class "HasoSlopes.lvclass">, "Phase out"=w905:refnum<class "Phase.lvclass">)  [unwired: 3 in]
                    n263 = local read "idxType"() -> (w893:enum16{"Wyant", "ANSI"})
                    n264 = call "slopes2zern.vi"("HasoSlopes in"=w900, "error in (no error)"=w899, "idxType"=w893) -> ("HasoSlopes out"=w897:refnum<class "HasoSlopes.lvclass">, "Zernike Coefficients"=w892:dbl[], "error out"=w898:errorcluster)  [unwired: 3 in, 2 out]
                    n265 = call <userlib>:"LVClass_Pupil ctor from HasoSlopes.vi"("Pupil in"=w904, "HasoSlopes.lvclass"=w891, "error in (no error)"=w898) -> ("Pupil out"=w915:refnum<class "Pupil.lvclass">, "error out"=w916:errorcluster)  [unwired: 11 in]
                    n266 = case shown="True" w896 {
                      tunnel: w895 -> [_ w925]
                      tunnel: w894 -> [_ w924]
                      tunnel: w892 -> [_ w923]
                      tunnel: w891 -> [_ w922]
                      frame False {
                      }
                      frame True {
                        n267 = stacked-sequence {
                          tunnel: w925 -> [w929 w935]
                          tunnel: w924 -> [w928 w934]
                          tunnel: w923 -> [_ w933]
                          tunnel: w922 -> [w926 _]
                          frame #0 {
                            n268 = Concatenate Strings(w929, "_slopesMeas", ".has") -> (w932:string)
                            n269 = Build Path(base path=w928, name or relative path=w932) -> (appended path=w927:path)
                            n270 = call <userlib>:"LVClass_HasoSlopes Save.vi"("HasoSlopes in"=w926, "path"=w927) -> ()  [unwired: 12 in, 2 out]
                          }
                          frame #1 {
                            n271 = Concatenate Strings(w935, "_zernCoefMeas", ".txt") -> (w938:string)
                            n272 = Build Path(base path=w934, name or relative path=w938) -> (appended path=w939:path)
                            n273 = Array To Spreadsheet String(array=w933, 3:"%f") -> (spreadsheet string=w940:string)  [unwired: 1 in]
                            n274 = Write to Text File(file (use dialog)=w939, text=w940) -> ()  [unwired: 2 in, 3 out]
                          }
                        }
                      }
                    }
                    n275 = call <userlib>:"LVClasse_Phase GetStatisticDatas.vi"("Phase in"=w905, "error in (no error)"=w916) -> ("Phase out"=w921:refnum<class "Phase.lvclass">, "StatisticsData"=w901:T2, "error out"=w919:errorcluster)  [unwired: 11 in]
                    n276 = local write "Phase statistics"(w901) -> ()
                    n277 = call <userlib>:"LVClasse_Phase Get Data.vi"("Phase in"=w921, "Pupil"=w915, "error in (no error)"=w919) -> ("Phase out"=w917:refnum<class "Phase.lvclass">, "data"=w902:sgl[][], "Pupil (dup)"=w918:refnum<class "Pupil.lvclass">, "error out"=w920:errorcluster)  [unwired: 9 in]
                    n278 = local write "Zernike Measured"(w892) -> ()
                    n279 = local write "Phase values"(w902) -> ()
                  }
                  frame Error {
                  }
                }
              }
            }
          }
          frame #3 {
            # "Apply offset to DM"
            n280 = case shown="True" w958 {
              tunnel: w961 -> [_ w969]
              tunnel: [w962 w963] -> w960
              tunnel: w959 -> [w962 w965]
              frame False {
              }
              frame True {
                # "Delay for DM response"
                n281 = local read "Initial offset"() -> (w968:bool)
                n282 = case shown="True" w968 {
                  tunnel: [w974 w979] -> w966
                  frame False {
                    n283 = Initialize Array(0.0, 52) -> (w974:dbl[])
                  }
                  frame True {
                    n284 = local read "Offset command file"() -> (w978:path)
                    n285 = call-poly <vilib>:"Read From Spreadsheet File.vi"("format (%.3f)"="%.8f", "file path (dialog if empty)"=w978) -> ("first row"=w979:dbl[])  [unwired: 5 in, 4 out]
                  }
                }
                n286 = local write "Initial Positions"(w966) -> ()
                n287 = call <userlib>:"LVClass_WavefrontCorrector Move to Absolute Position.vi"("WavefrontCorrector in"=w969, "Absolute Positions"=w966, "error in (no error)"=w965) -> ("WavefrontCorrector out"=w970:refnum<class "WavefrontCorrector.lvclass">, "error out"=w971:errorcluster)  [unwired: 11 in]
                n288 = call <userlib>:"LVClass_WavefrontCorrector Get Current Position.vi"("WavefrontCorrector in"=w970, "error in (no error)"=w971) -> ("Wavefront Corrector Position"=w967:T14, "error out"=w964:errorcluster)  [unwired: 11 in, 1 out]
                n289 = local write "Initial Positions"(w967) -> ()
                n290 = flat-sequence {
                  tunnel: [w972] -> w963
                  tunnel: w964 -> [w972]
                  frame #0 {
                    n291 = Wait (ms)(milliseconds to wait=u32 50) -> ()  [unwired: 1 out]
                  }
                }
              }
            }
          }
          frame #4 {
            n292 = case shown="True" w982 {
              tunnel: w993 -> [_ w1008]
              tunnel: w992 -> [_ w1007]
              tunnel: w991 -> [_ w1006]
              tunnel: w990 -> [_ w1005]
              tunnel: w989 -> [_ w1004]
              tunnel: w981 -> [w994 w1003]
              tunnel: w988 -> [_ w1002]
              tunnel: w987 -> [_ w1001]
              tunnel: w986 -> [_ w1000]
              tunnel: w985 -> [w995 w998]
              tunnel: [w995 w997] -> w983
              tunnel: [w994 w996] -> w980
              frame False {
              }
              frame True {
                n293 = local read "HASO ready"() -> (w999:bool)
                n294 = case shown="True" w999 {
                  tunnel: w1008 -> [_ w1036]
                  tunnel: w1006 -> [_ w1035]
                  tunnel: w1005 -> [_ w1034]
                  tunnel: [w1009 w1031] -> w997
                  tunnel: w1007 -> [_ w1029]
                  tunnel: w1000 -> [_ w1014]
                  tunnel: w998 -> [w1009 w1015]
                  tunnel: w1003 -> [w1012 w1017]
                  tunnel: w1002 -> [w1011 w1028]
                  tunnel: [w1012 w1019] -> w996
                  tunnel: [w1011 w1027] -> _
                  tunnel: w1004 -> [w1013 w1026]
                  tunnel: w1001 -> [w1010 w1025]
                  tunnel: [w1013 w1024] -> _
                  tunnel: [w1010 w1023] -> _
                  frame False {
                  }
                  frame True {
                    n295 = property on="nb_images (set)" class="DigNum (strict)"() -> ("Value"=w1037:u32)  [unwired: 2 in, 2 out]
                    n296 = case shown="2, Default" w1037 {
                      tunnel: [w1117 w1119] -> w1038
                      tunnel: w1029 -> [w1116 _]
                      tunnel: w1036 -> [w1117 _]
                      tunnel: [w1116 w1118] -> w1033
                      tunnel: w1035 -> [_ w1119]
                      tunnel: w1034 -> [_ w1118]
                      frame 2, Default {
                      }
                      frame 1 {
                      }
                    }
                    n297 = call <userlib>:"LVClass_Camera get image.vi"("Camera in"=w1014, "Image"=w1038, "Image RAW"=w1033, "remove_background"=FALSE, "error in (no error)"=w1015) -> ("Image (dup)"=w1032:refnum<class "Image.lvclass">, "error out"=w1030:errorcluster)  [unwired: 7 in, 2 out]
                    n298 = case shown="No Error" w1030 {
                      selector: w1030 -> [w1113 w1114]
                      tunnel: w1032 -> [w1110 w1115]
                      tunnel: [w1109 w1115] -> w1022
                      tunnel: [w1108 w1114] -> w1021
                      frame No Error {
                        # "get image"
                        n299 = call <userlib>:"LVClass_Image get image data.vi"("Image in"=w1110, "error in (no error)"=w1113) -> ("Image out"=w1112:refnum<class "Image.lvclass">, "Image data out"=w1107:u32[][], "error out"=w1111:errorcluster)  [unwired: 11 in]
                        n300 = call <userlib>:"LVClass_Image get image information.vi"("Image in"=w1112, "error in (no error)"=w1111) -> ("Image out"=w1109:refnum<class "Image.lvclass">, "error out"=w1108:errorcluster)  [unwired: 11 in, 1 out]
                        n301 = local write "HASO intensity"(w1107) -> ()
                      }
                      frame Error {
                      }
                    }
                    n302 = case shown="No Error" w1021 {
                      selector: w1021 -> [w1065 w1106]
                      tunnel: [w1071 w1106] -> w1031
                      tunnel: w1022 -> [w1064 _]
                      tunnel: [w1069 w1103] -> w1023
                      tunnel: [w1068 w1105] -> w1024
                      tunnel: refnum<class "HasoSlopes.lvclass"> refnum ("HasoSlopes in") -> [w1061 w1102]
                      tunnel: w1028 -> [w1060 w1104]
                      tunnel: [w1059 w1104] -> w1027
                      tunnel: w1026 -> [w1058 w1105]
                      tunnel: w1025 -> [w1056 w1103]
                      tunnel: [w1041 w1101] -> w1019
                      tunnel: [w1039 w1102] -> w1018
                      tunnel: w1017 -> [w1040 w1101]
                      frame No Error {
                        # "phaseout"
                        n303 = local read "File Base Name"() -> (w1048:string)
                        n304 = local read "Save File"() -> (w1049:bool)
                        n305 = local read "Output path"() -> (w1047:path)
                        n306 = call "image2slopes.vi"("error in (no error)"=w1065, "Image in"=w1064, "HasoEngine in"=w1060, "HasoSlopes in"=w1061) -> ("error out"=w1043:errorcluster, "HasoEngine out"=w1059:refnum<class "HasoEngine.lvclass">, "HasoSlopes out"=w1039:refnum<class "HasoSlopes.lvclass">)  [unwired: 4 in, 1 out]
                        n307 = local read "Filter"() -> (w1055:u8[])
                        n308 = call <userlib>:"LVClass_HasoSlopes Apply Substractor.vi"("HasoSlopes in"=w1040, "HasoSlopes to substract"=w1039, "error in (no error)"=w1043) -> ("HasoSlopes out"=w1044:refnum<class "HasoSlopes.lvclass">, "error out"=w1042:errorcluster)  [unwired: 11 in]
                        n309 = call "slopes2phase.vi"("TypePhase"=WavefrontReconstructionMode."Modal_Zernike", "Number of coefficients"=u8 32, "error in (no error)"=w1042, "Filter"=w1055, "HasoSlopes in"=w1044, "Phase in"=w1058) -> ("error out"=w1051:errorcluster, "HasoSlopes out"=w1052:refnum<class "HasoSlopes.lvclass">, "Phase out"=w1057:refnum<class "Phase.lvclass">)  [unwired: 3 in]
                        n310 = local read "idxType"() -> (w1046:enum16{"Wyant", "ANSI"})
                        n311 = call "slopes2zern.vi"("HasoSlopes in"=w1052, "error in (no error)"=w1051, "idxType"=w1046) -> ("HasoSlopes out"=w1041:refnum<class "HasoSlopes.lvclass">, "Zernike Coefficients"=w1045:dbl[], "error out"=w1050:errorcluster)  [unwired: 3 in, 2 out]
                        n312 = call <userlib>:"LVClass_Pupil ctor from HasoSlopes.vi"("Pupil in"=w1056, "HasoSlopes.lvclass"=w1044, "error in (no error)"=w1050) -> ("Pupil out"=w1066:refnum<class "Pupil.lvclass">, "error out"=w1067:errorcluster)  [unwired: 11 in]
                        n313 = case shown="True" w1049 {
                          tunnel: w1048 -> [_ w1077]
                          tunnel: w1047 -> [_ w1076]
                          tunnel: w1045 -> [_ w1075]
                          tunnel: w1044 -> [_ w1073]
                          tunnel: w1039 -> [_ w1074]
                          frame False {
                          }
                          frame True {
                            n314 = stacked-sequence {
                              tunnel: w1077 -> [w1081 w1088 w1094]
                              tunnel: w1076 -> [w1080 w1087 w1093]
                              tunnel: w1075 -> [_ _ w1092]
                              tunnel: w1074 -> [w1078 _ _]
                              tunnel: w1073 -> [_ w1085 _]
                              frame #0 {
                                n315 = Concatenate Strings(w1081, "_slopesOffset", ".has") -> (w1084:string)
                                n316 = Build Path(base path=w1080, name or relative path=w1084) -> (appended path=w1079:path)
                                n317 = call <userlib>:"LVClass_HasoSlopes Save.vi"("HasoSlopes in"=w1078, "path"=w1079) -> ()  [unwired: 12 in, 2 out]
                              }
                              frame #1 {
                                n318 = Concatenate Strings(w1088, "_slopesNet", ".has") -> (w1091:string)
                                n319 = Build Path(base path=w1087, name or relative path=w1091) -> (appended path=w1086:path)
                                n320 = call <userlib>:"LVClass_HasoSlopes Save.vi"("HasoSlopes in"=w1085, "path"=w1086) -> ()  [unwired: 12 in, 2 out]
                              }
                              frame #2 {
                                n321 = Concatenate Strings(w1094, "_zernCoefNet", ".txt") -> (w1097:string)
                                n322 = Build Path(base path=w1093, name or relative path=w1097) -> (appended path=w1098:path)
                                n323 = Array To Spreadsheet String(array=w1092, 3:"%f") -> (spreadsheet string=w1099:string)  [unwired: 1 in]
                                n324 = Write to Text File(file (use dialog)=w1098, text=w1099) -> ()  [unwired: 2 in, 3 out]
                              }
                            }
                          }
                        }
                        n325 = call <userlib>:"LVClasse_Phase GetStatisticDatas.vi"("Phase in"=w1057, "error in (no error)"=w1067) -> ("Phase out"=w1072:refnum<class "Phase.lvclass">, "StatisticsData"=w1053:T2, "error out"=w1070:errorcluster)  [unwired: 11 in]
                        n326 = local write "Phase statistics"(w1053) -> ()
                        n327 = call <userlib>:"LVClasse_Phase Get Data.vi"("Phase in"=w1072, "Pupil"=w1066, "error in (no error)"=w1070) -> ("Phase out"=w1068:refnum<class "Phase.lvclass">, "data"=w1054:sgl[][], "Pupil (dup)"=w1069:refnum<class "Pupil.lvclass">, "error out"=w1071:errorcluster)  [unwired: 9 in]
                        n328 = local write "Zernike Measured"(w1045) -> ()
                        n329 = local write "Phase values"(w1054) -> ()
                      }
                      frame Error {
                      }
                    }
                    n330 = call <userlib>:"LVClass_HasoSlopes dtor.vi"("HasoSlopes in"=w1018) -> ()  [unwired: 13 in, 2 out]
                  }
                }
              }
            }
            n331 = Unbundle By Name(w983) -> ("status"=w984:bool)
          }
        }
      }
      event "Record Batch": Mouse Up {
        n332 = event-data() -> ()  [unwired: 1 in, 8 out]
        n333 = local read "Idx start"() -> (w1120:u32)
        n334 = local read "Idx end"() -> (w1121:u32)
        n335 = Subtract(x=w1121, y=w1120) -> (x-y=w1122:u32)
        n336 = Increment(x=w1122) -> (x+1=w1123:u32)
        n337 = for {
          N: w1123 -> [_]
          tunnel: [w1162] -> w1141
          tunnel: w1135 -> [w1157]
          tunnel: w1134 -> [w1156]
          tunnel: w1133 -> [w1155]
          tunnel: w1132 -> [w1154]
          tunnel: w1129 -> [w1151]
          tunnel: w1128 -> [w1150]
          shift-right: [w1160] -> w1139
          shift-left: w1140 -> [w1161]
          shift-right: [w1158] -> w1136
          shift-left: w1138 -> [w1159]
          shift-right: [w1148] -> w1126
          shift-left: w1131 -> [w1153]
          shift-right: [w1149] -> w1127
          shift-left: w1130 -> [w1152]
          shift-right: [w1146] -> w1124
          shift-left: w1125 -> [w1147]
          tunnel: w1120 -> [w1143]
          i -> [w1144]
          n338 = Add(x=w1143, y=w1144) -> (x+y=w1142:u32)
          n339 = local read "Net Rp"() -> (w1145:bool)
          n340 = stacked-sequence {
            seq-local: [_ _ _ w1450 _] -> [_ _ _ _ w1475]
            seq-local: [_ _ w1337 _ _] -> [_ _ _ w1449 _]
            seq-local: [_ w1206 _ _ _] -> [_ _ w1338 _ _]
            seq-local: [_ _ w1336 _ _] -> [_ _ _ _ w1471]
            tunnel: [_ _ _ _ w1474] -> w1162
            tunnel: w1161 -> [_ w1219 _ _ _]
            tunnel: [_ _ _ _ w1473] -> w1160
            tunnel: w1159 -> [_ w1218 _ w1451 _]
            tunnel: [_ w1216 _ _ _] -> w1158
            tunnel: w1157 -> [_ _ w1350 _ w1483]
            tunnel: w1156 -> [_ _ w1349 _ w1482]
            tunnel: w1155 -> [_ _ w1348 _ w1481]
            tunnel: w1154 -> [_ _ w1347 _ w1480]
            tunnel: w1153 -> [_ _ w1346 _ w1479]
            tunnel: w1152 -> [_ _ w1345 _ _]
            tunnel: w1151 -> [_ _ w1344 _ w1478]
            tunnel: w1147 -> [_ _ w1343 _ w1477]
            tunnel: w1150 -> [_ _ w1342 _ w1476]
            tunnel: [_ _ _ _ w1470] -> w1149
            tunnel: [_ _ w1340 _ _] -> w1148
            tunnel: [_ _ w1339 _ _] -> w1146
            tunnel: w1145 -> [_ _ _ w1448 w1472]
            tunnel: w1142 -> [w1164 w1207 _ _ _]
            frame #0 {
              # "Create output folder path"
              n341 = Get Date/Time In Seconds() -> (seconds since 1Jan1904=w1185:timestamp)
              n342 = local read "Folder Name"() -> (w1177:string)
              n343 = local read "idxType"() -> (w1168:enum16{"Wyant", "ANSI"})
              n344 = Number To Decimal String(number=w1164) -> (decimal integer string=w1165:string)  [unwired: 1 in]
              n345 = Format Date/Time String(time format string (%c)="%Y%m%d", seconds (now)=w1185) -> (date/time string=w1184:string)  [unwired: 1 in]
              n346 = local read "Main Path"() -> (w1178:path)
              n347 = case shown="\"ANSI\"" w1168 {
                tunnel: ["Wyant" "ANSI"] -> w1167
                frame "Wyant", Default {
                }
                frame "ANSI" {
                }
              }
              n348 = local read "Subfolder"() -> (w1176:string)
              n349 = Concatenate Strings(w1184, "_", w1177) -> (w1183:string)
              n350 = Build Path(base path=w1178, name or relative path=w1183) -> (appended path=w1181:path)
              n351 = call <vilib>:"Check if File or Folder Exists.vi"("path"=w1181) -> ("error out"=w1174:errorcluster, "file or folder exists?"=w1187:bool)  [unwired: 8 in, 1 out]
              n352 = Concatenate Strings(w1167, "_idx_", w1165) -> (w1163:string)
              n353 = Build Path(base path=w1181, name or relative path=w1176) -> (appended path=w1172:path)
              n354 = Build Path(base path=w1172, name or relative path=w1163) -> (appended path=w1169:path)
              n355 = local write "Current status"(w1163) -> ()
              n356 = case shown="False" w1187 {
                tunnel: w1181 -> [w1203 _]
                tunnel: w1174 -> [w1202 w1204]
                tunnel: [w1201 w1204] -> w1173
                frame False {
                  n357 = Create Folder(path (use dialog)=w1203, error in=w1202) -> (error out=w1201:errorcluster)  [unwired: 1 in, 2 out]
                }
                frame True {
                }
              }
              n358 = call <vilib>:"Check if File or Folder Exists.vi"("error in (no error)"=w1173, "path"=w1172) -> ("error out"=w1171:errorcluster, "file or folder exists?"=w1175:bool)  [unwired: 7 in, 1 out]
              n359 = case shown="True" w1175 {
                tunnel: w1172 -> [w1192 _]
                tunnel: w1171 -> [w1191 w1193]
                tunnel: [w1190 w1193] -> w1170
                frame False {
                  n360 = Create Folder(path (use dialog)=w1192, error in=w1191) -> (error out=w1190:errorcluster)  [unwired: 1 in, 2 out]
                }
                frame True {
                }
              }
              n361 = call <vilib>:"Check if File or Folder Exists.vi"("error in (no error)"=w1170, "path"=w1169) -> ("error out"=w1182:errorcluster, "file or folder exists?"=w1186:bool)  [unwired: 7 in, 1 out]
              n362 = case shown="False" w1186 {
                tunnel: w1169 -> [w1195 w1199]
                tunnel: w1182 -> [w1194 w1200]
                frame False {
                  n363 = Create Folder(path (use dialog)=w1195, error in=w1194) -> ()  [unwired: 1 in, 3 out]
                }
                frame True {
                  n364 = Delete(path (use dialog)=w1199, entire hierarchy (F)=TRUE, error in=w1200) -> (deleted path=w1197:path, error out=w1196:errorcluster)  [unwired: 2 in, 1 out]
                  n365 = Create Folder(path (use dialog)=w1197, error in=w1196) -> ()  [unwired: 1 in, 3 out]
                }
              }
              n366 = local write "Output path"(w1169) -> ()
            }
            frame #1 {
              # "Delay for DM response"
              # "Apply command to DM"
              n367 = local read "Initial offset"() -> (w1217:bool)
              n368 = case shown="True" w1217 {
                tunnel: [w1305 w1310] -> w1208
                frame False {
                  n369 = Initialize Array(0.0, 52) -> (w1305:dbl[])
                }
                frame True {
                  n370 = local read "Offset command file"() -> (w1309:path)
                  n371 = call-poly <vilib>:"Read From Spreadsheet File.vi"("format (%.3f)"="%.8f", "file path (dialog if empty)"=w1309) -> ("first row"=w1310:dbl[])  [unwired: 5 in, 4 out]
                }
              }
              n372 = local read "Additional Command"() -> (w1223:bool)
              n373 = case shown="True" w1223 {
                tunnel: [w1312 w1335] -> w1209
                tunnel: [w1311 w1334] -> w1220
                tunnel: w1219 -> [w1311 w1333]
                tunnel: w1207 -> [_ w1316]
                frame False {
                  n374 = Initialize Array(0.0, 52) -> (w1312:dbl[])
                }
                frame True {
                  w1317 = 1
                  n375 = local read "Coef value"() -> (w1319:dbl)
                  n376 = local read "Initial haso file"() -> (w1323:path)
                  n377 = Initialize Array(w1316, w1317) -> (w1315:u32[])
                  n378 = Initialize Array(w1319, w1317) -> (w1318:dbl[])
                  n379 = local read "Haso configuration file"() -> (w1324:path)
                  n380 = local read "interaction matrix file"() -> (w1322:path)
                  n381 = local read "idxType"() -> (w1325:enum16{"Wyant", "ANSI"})
                  n382 = call "zern2command.vi"("Haso configuration file"=w1324, "idxType"=w1325, "interaction matrix file"=w1322, "error in (no error)"=w1333, "Zern coef in"=w1318, "Zern index in"=w1315, "Initial haso file"=w1323) -> ("error out"=w1326:errorcluster, "Offset Positions"=w1335:sgl[], "Zern pupil out"=w1327:refnum<class "Pupil.lvclass">, "ModalCoef out"=w1328:refnum<class "ModalCoef.lvclass">)  [unwired: 1 in]
                  n383 = call <userlib>:"LVClass_ModalCoef GetData.vi"("ModalCoef in"=w1328, "Pupil.lvclass"=w1327, "error in (no error)"=w1326) -> ("ModalCoef out"=w1332:refnum<class "ModalCoef.lvclass">, "coef"=w1321:sgl[], "index"=w1320:u32[], "Pupil.lvclass (dup)"=w1331:refnum<class "Pupil.lvclass">, "error out"=w1330:errorcluster)  [unwired: 8 in]
                  n384 = local write "Zern index out"(w1320) -> ()
                  n385 = call <userlib>:"LVClass_Pupil dtor.vi"("Pupil in"=w1331, "error in (no error)"=w1330) -> ("error out"=w1329:errorcluster)  [unwired: 12 in, 1 out]
                  n386 = local write "Zern coef out"(w1321) -> ()
                  n387 = call <userlib>:"LVClass_ModalCoef dtor.vi"("ModalCoef in"=w1332, "error in (no error)"=w1329) -> ("error out"=w1334:errorcluster)  [unwired: 12 in, 1 out]
                }
              }
              n388 = local read "File Base Name"() -> (w1210:string)
              n389 = local read "Output path"() -> (w1214:path)
              n390 = local read "Input type"() -> (w1211:T4)
              n391 = local read "Save File"() -> (w1215:bool)
              n392 = local write "Initial Positions"(w1208) -> ()
              n393 = Add(x=w1209, y=w1208) -> (x+y=w1212:dbl[])
              n394 = call <userlib>:"LVClass_WavefrontCorrector Move to Absolute Position.vi"("WavefrontCorrector in"=w1218, "Absolute Positions"=w1212, "error in (no error)"=w1220) -> ("WavefrontCorrector out"=w1221:refnum<class "WavefrontCorrector.lvclass">, "error out"=w1222:errorcluster)  [unwired: 11 in]
              n395 = call <userlib>:"LVClass_WavefrontCorrector Get Current Position.vi"("WavefrontCorrector in"=w1221, "error in (no error)"=w1222) -> ("WavefrontCorrector out"=w1216:refnum<class "WavefrontCorrector.lvclass">, "Wavefront Corrector Position"=w1213:T14, "error out"=w1205:errorcluster)  [unwired: 11 in]
              n396 = case shown="True" w1215 {
                tunnel: w1214 -> [_ w1232]
                tunnel: w1210 -> [_ w1231]
                tunnel: w1208 -> [_ w1230]
                tunnel: w1209 -> [_ w1229]
                tunnel: w1212 -> [_ w1228]
                tunnel: w1211 -> [_ w1227]
                tunnel: w1213 -> [_ w1226]
                frame False {
                }
                frame True {
                  n397 = stacked-sequence {
                    tunnel: w1232 -> [w1237 w1246 w1255 w1264 w1271 w1283 w1295]
                    tunnel: w1231 -> [w1235 w1244 w1253 w1262 w1270 w1282 w1294]
                    tunnel: w1230 -> [w1233 _ _ _ _ _ _]
                    tunnel: w1229 -> [_ w1242 _ _ _ _ _]
                    tunnel: w1228 -> [_ _ w1251 _ _ _ _]
                    tunnel: w1227 -> [_ _ _ _ w1269 w1281 w1293]
                    tunnel: w1226 -> [_ _ _ w1260 _ _ _]
                    frame #0 {
                      n398 = Concatenate Strings(w1235, "_cmdOffset", ".dat") -> (w1238:string)
                      n399 = Build Path(base path=w1237, name or relative path=w1238) -> (appended path=w1239:path)
                      n400 = Array To Spreadsheet String(array=w1233, 3:"%f") -> (spreadsheet string=w1240:string)  [unwired: 1 in]
                      n401 = Write to Text File(file (use dialog)=w1239, text=w1240) -> ()  [unwired: 2 in, 3 out]
                    }
                    frame #1 {
                      n402 = Concatenate Strings(w1244, "_cmdAdd", ".dat") -> (w1247:string)
                      n403 = Build Path(base path=w1246, name or relative path=w1247) -> (appended path=w1248:path)
                      n404 = Array To Spreadsheet String(array=w1242, 3:"%f") -> (spreadsheet string=w1249:string)  [unwired: 1 in]
                      n405 = Write to Text File(file (use dialog)=w1248, text=w1249) -> ()  [unwired: 2 in, 3 out]
                    }
                    frame #2 {
                      n406 = Concatenate Strings(w1253, "_cmdFinal", ".dat") -> (w1256:string)
                      n407 = Build Path(base path=w1255, name or relative path=w1256) -> (appended path=w1257:path)
                      n408 = Array To Spreadsheet String(array=w1251, 3:"%f") -> (spreadsheet string=w1258:string)  [unwired: 1 in]
                      n409 = Write to Text File(file (use dialog)=w1257, text=w1258) -> ()  [unwired: 2 in, 3 out]
                    }
                    frame #3 {
                      n410 = Concatenate Strings(w1262, "_cmdFinalMirror", ".dat") -> (w1265:string)
                      n411 = Build Path(base path=w1264, name or relative path=w1265) -> (appended path=w1266:path)
                      n412 = Array To Spreadsheet String(array=w1260, 3:"%f") -> (spreadsheet string=w1267:string)  [unwired: 1 in]
                      n413 = Write to Text File(file (use dialog)=w1266, text=w1267) -> ()  [unwired: 2 in, 3 out]
                    }
                    frame #4 {
                      n414 = case shown="\"Zernike Coef\", Default" w1269 {
                        tunnel: w1271 -> [_ w1276]
                        tunnel: w1270 -> [_ w1274]
                        frame "Zero Input" {
                        }
                        frame "Zernike Coef", Default {
                          n415 = local read "Zern coef in"() -> (w1272:sgl[])
                          n416 = Concatenate Strings(w1274, "_zernCoef", ".txt") -> (w1277:string)
                          n417 = Build Path(base path=w1276, name or relative path=w1277) -> (appended path=w1278:path)
                          n418 = Array To Spreadsheet String(array=w1272, 3:"%f") -> (spreadsheet string=w1279:string)  [unwired: 1 in]
                          n419 = Write to Text File(file (use dialog)=w1278, text=w1279) -> ()  [unwired: 2 in, 3 out]
                        }
                      }
                    }
                    frame #5 {
                      n420 = case shown="\"Zernike Coef\", Default" w1281 {
                        tunnel: w1283 -> [_ w1288]
                        tunnel: w1282 -> [_ w1286]
                        frame "Zero Input" {
                        }
                        frame "Zernike Coef", Default {
                          n421 = local read "Zern index in"() -> (w1284:i32[])
                          n422 = Concatenate Strings(w1286, "_zernIdx", ".txt") -> (w1289:string)
                          n423 = Build Path(base path=w1288, name or relative path=w1289) -> (appended path=w1290:path)
                          n424 = Array To Spreadsheet String(array=w1284, 3:"%d") -> (spreadsheet string=w1291:string)  [unwired: 1 in]
                          n425 = Write to Text File(file (use dialog)=w1290, text=w1291) -> ()  [unwired: 2 in, 3 out]
                        }
                      }
                    }
                    frame #6 {
                      n426 = case shown="\"Zernike Coef\", Default" w1293 {
                        tunnel: w1295 -> [_ w1300]
                        tunnel: w1294 -> [_ w1298]
                        frame "Zero Input" {
                        }
                        frame "Zernike Coef", Default {
                          n427 = Concatenate Strings(w1298, "_zernCoefWyant", ".txt") -> (w1301:string)
                          n428 = local read "Zern coef out"() -> (w1296:sgl[])
                          n429 = Build Path(base path=w1300, name or relative path=w1301) -> (appended path=w1302:path)
                          n430 = Array To Spreadsheet String(array=w1296, 3:"%f") -> (spreadsheet string=w1303:string)  [unwired: 1 in]
                          n431 = Write to Text File(file (use dialog)=w1302, text=w1303) -> ()  [unwired: 2 in, 3 out]
                        }
                      }
                    }
                  }
                }
              }
              n432 = local write "Final Positions"(w1212) -> ()
              n433 = local write "DM Actuator Values"(w1213) -> ()
              n434 = flat-sequence {
                tunnel: [w1224] -> w1206
                tunnel: w1205 -> [w1224]
                frame #0 {
                  n435 = Wait (ms)(milliseconds to wait=u32 50) -> ()  [unwired: 1 out]
                }
              }
            }
            frame #2 {
              n436 = local read "HASO ready"() -> (w1341:bool)
              n437 = case shown="True" w1341 {
                tunnel: w1350 -> [_ w1376]
                tunnel: w1348 -> [_ w1375]
                tunnel: w1347 -> [_ w1374]
                tunnel: [w1351 w1371] -> w1337
                tunnel: w1349 -> [_ w1369]
                tunnel: w1342 -> [_ w1356]
                tunnel: w1338 -> [w1351 w1357]
                tunnel: w1345 -> [w1354 w1368]
                tunnel: w1344 -> [w1353 w1367]
                tunnel: [w1354 w1366] -> w1336
                tunnel: [w1353 w1365] -> _
                tunnel: w1346 -> [w1355 w1364]
                tunnel: w1343 -> [w1352 w1363]
                tunnel: [w1355 w1362] -> w1340
                tunnel: [w1352 w1361] -> w1339
                frame False {
                }
                frame True {
                  n438 = property on="nb_images (set)" class="DigNum (strict)"() -> ("Value"=w1377:u32)  [unwired: 2 in, 2 out]
                  n439 = case shown="2, Default" w1377 {
                    tunnel: [w1445 w1447] -> w1378
                    tunnel: w1369 -> [w1444 _]
                    tunnel: w1376 -> [w1445 _]
                    tunnel: [w1444 w1446] -> w1373
                    tunnel: w1375 -> [_ w1447]
                    tunnel: w1374 -> [_ w1446]
                    frame 2, Default {
                    }
                    frame 1 {
                    }
                  }
                  n440 = call <userlib>:"LVClass_Camera get image.vi"("Camera in"=w1356, "Image"=w1378, "Image RAW"=w1373, "remove_background"=FALSE, "error in (no error)"=w1357) -> ("Image (dup)"=w1372:refnum<class "Image.lvclass">, "error out"=w1370:errorcluster)  [unwired: 7 in, 2 out]
                  n441 = case shown="No Error" w1370 {
                    selector: w1370 -> [w1441 w1442]
                    tunnel: w1372 -> [w1438 w1443]
                    tunnel: [w1437 w1443] -> w1360
                    tunnel: [w1436 w1442] -> w1359
                    frame No Error {
                      # "get image"
                      n442 = call <userlib>:"LVClass_Image get image data.vi"("Image in"=w1438, "error in (no error)"=w1441) -> ("Image out"=w1440:refnum<class "Image.lvclass">, "Image data out"=w1435:u32[][], "error out"=w1439:errorcluster)  [unwired: 11 in]
                      n443 = call <userlib>:"LVClass_Image get image information.vi"("Image in"=w1440, "error in (no error)"=w1439) -> ("Image out"=w1437:refnum<class "Image.lvclass">, "error out"=w1436:errorcluster)  [unwired: 11 in, 1 out]
                      n444 = local write "HASO intensity"(w1435) -> ()
                    }
                    frame Error {
                    }
                  }
                  n445 = case shown="No Error" w1359 {
                    selector: w1359 -> [w1402 w1434]
                    tunnel: [w1408 w1434] -> w1371
                    tunnel: w1360 -> [w1401 _]
                    tunnel: [w1406 w1430] -> w1361
                    tunnel: [w1405 w1433] -> w1362
                    tunnel: w1368 -> [w1398 w1432]
                    tunnel: w1367 -> [w1397 w1431]
                    tunnel: [w1385 w1432] -> w1366
                    tunnel: [w1396 w1431] -> w1365
                    tunnel: w1364 -> [w1394 w1433]
                    tunnel: w1363 -> [w1392 w1430]
                    frame No Error {
                      # "phaseout"
                      n446 = local read "File Base Name"() -> (w1383:string)
                      n447 = local read "Save File"() -> (w1384:bool)
                      n448 = local read "Output path"() -> (w1382:path)
                      n449 = call "image2slopes.vi"("error in (no error)"=w1402, "Image in"=w1401, "HasoEngine in"=w1397, "HasoSlopes in"=w1398) -> ("error out"=w1395:errorcluster, "HasoEngine out"=w1396:refnum<class "HasoEngine.lvclass">, "HasoSlopes out"=w1379:refnum<class "HasoSlopes.lvclass">)  [unwired: 4 in, 1 out]
                      n450 = local read "Filter"() -> (w1391:u8[])
                      n451 = call "slopes2phase.vi"("TypePhase"=WavefrontReconstructionMode."Modal_Zernike", "Number of coefficients"=u8 32, "error in (no error)"=w1395, "Filter"=w1391, "HasoSlopes in"=w1379, "Phase in"=w1394) -> ("error out"=w1387:errorcluster, "HasoSlopes out"=w1388:refnum<class "HasoSlopes.lvclass">, "Phase out"=w1393:refnum<class "Phase.lvclass">)  [unwired: 3 in]
                      n452 = local read "idxType"() -> (w1381:enum16{"Wyant", "ANSI"})
                      n453 = call "slopes2zern.vi"("HasoSlopes in"=w1388, "error in (no error)"=w1387, "idxType"=w1381) -> ("HasoSlopes out"=w1385:refnum<class "HasoSlopes.lvclass">, "Zernike Coefficients"=w1380:dbl[], "error out"=w1386:errorcluster)  [unwired: 3 in, 2 out]
                      n454 = call <userlib>:"LVClass_Pupil ctor from HasoSlopes.vi"("Pupil in"=w1392, "HasoSlopes.lvclass"=w1379, "error in (no error)"=w1386) -> ("Pupil out"=w1403:refnum<class "Pupil.lvclass">, "error out"=w1404:errorcluster)  [unwired: 11 in]
                      n455 = case shown="True" w1384 {
                        tunnel: w1383 -> [_ w1413]
                        tunnel: w1382 -> [_ w1412]
                        tunnel: w1380 -> [_ w1411]
                        tunnel: w1379 -> [_ w1410]
                        frame False {
                        }
                        frame True {
                          n456 = stacked-sequence {
                            tunnel: w1413 -> [w1417 w1423]
                            tunnel: w1412 -> [w1416 w1422]
                            tunnel: w1411 -> [_ w1421]
                            tunnel: w1410 -> [w1414 _]
                            frame #0 {
                              n457 = Concatenate Strings(w1417, "_slopesMeas", ".has") -> (w1420:string)
                              n458 = Build Path(base path=w1416, name or relative path=w1420) -> (appended path=w1415:path)
                              n459 = call <userlib>:"LVClass_HasoSlopes Save.vi"("HasoSlopes in"=w1414, "path"=w1415) -> ()  [unwired: 12 in, 2 out]
                            }
                            frame #1 {
                              n460 = Concatenate Strings(w1423, "_zernCoefMeas", ".txt") -> (w1426:string)
                              n461 = Build Path(base path=w1422, name or relative path=w1426) -> (appended path=w1427:path)
                              n462 = Array To Spreadsheet String(array=w1421, 3:"%f") -> (spreadsheet string=w1428:string)  [unwired: 1 in]
                              n463 = Write to Text File(file (use dialog)=w1427, text=w1428) -> ()  [unwired: 2 in, 3 out]
                            }
                          }
                        }
                      }
                      n464 = call <userlib>:"LVClasse_Phase GetStatisticDatas.vi"("Phase in"=w1393, "error in (no error)"=w1404) -> ("Phase out"=w1409:refnum<class "Phase.lvclass">, "StatisticsData"=w1389:T2, "error out"=w1407:errorcluster)  [unwired: 11 in]
                      n465 = local write "Phase statistics"(w1389) -> ()
                      n466 = call <userlib>:"LVClasse_Phase Get Data.vi"("Phase in"=w1409, "Pupil"=w1403, "error in (no error)"=w1407) -> ("Phase out"=w1405:refnum<class "Phase.lvclass">, "data"=w1390:sgl[][], "Pupil (dup)"=w1406:refnum<class "Pupil.lvclass">, "error out"=w1408:errorcluster)  [unwired: 9 in]
                      n467 = local write "Zernike Measured"(w1380) -> ()
                      n468 = local write "Phase values"(w1390) -> ()
                    }
                    frame Error {
                    }
                  }
                }
              }
            }
            frame #3 {
              # "Apply offset to DM"
              n469 = case shown="True" w1448 {
                tunnel: w1451 -> [_ w1459]
                tunnel: [w1452 w1454] -> w1450
                tunnel: w1449 -> [w1452 w1455]
                frame False {
                }
                frame True {
                  # "Delay for DM response"
                  n470 = local read "Initial offset"() -> (w1458:bool)
                  n471 = case shown="True" w1458 {
                    tunnel: [w1464 w1469] -> w1456
                    frame False {
                      n472 = Initialize Array(0.0, 52) -> (w1464:dbl[])
                    }
                    frame True {
                      n473 = local read "Offset command file"() -> (w1468:path)
                      n474 = call-poly <vilib>:"Read From Spreadsheet File.vi"("format (%.3f)"="%.8f", "file path (dialog if empty)"=w1468) -> ("first row"=w1469:dbl[])  [unwired: 5 in, 4 out]
                    }
                  }
                  n475 = local write "Initial Positions"(w1456) -> ()
                  n476 = call <userlib>:"LVClass_WavefrontCorrector Move to Absolute Position.vi"("WavefrontCorrector in"=w1459, "Absolute Positions"=w1456, "error in (no error)"=w1455) -> ("WavefrontCorrector out"=w1460:refnum<class "WavefrontCorrector.lvclass">, "error out"=w1461:errorcluster)  [unwired: 11 in]
                  n477 = call <userlib>:"LVClass_WavefrontCorrector Get Current Position.vi"("WavefrontCorrector in"=w1460, "error in (no error)"=w1461) -> ("Wavefront Corrector Position"=w1457:T14, "error out"=w1453:errorcluster)  [unwired: 11 in, 1 out]
                  n478 = local write "Initial Positions"(w1457) -> ()
                  n479 = flat-sequence {
                    tunnel: [w1462] -> w1454
                    tunnel: w1453 -> [w1462]
                    frame #0 {
                      n480 = Wait (ms)(milliseconds to wait=u32 50) -> ()  [unwired: 1 out]
                    }
                  }
                }
              }
            }
            frame #4 {
              n481 = case shown="True" w1472 {
                tunnel: w1483 -> [_ w1498]
                tunnel: w1482 -> [_ w1497]
                tunnel: w1481 -> [_ w1496]
                tunnel: w1480 -> [_ w1495]
                tunnel: w1479 -> [_ w1494]
                tunnel: w1471 -> [w1484 w1493]
                tunnel: w1478 -> [_ w1492]
                tunnel: w1477 -> [_ w1491]
                tunnel: w1476 -> [_ w1490]
                tunnel: w1475 -> [w1485 w1488]
                tunnel: [w1485 w1487] -> w1473
                tunnel: [w1484 w1486] -> w1470
                frame False {
                }
                frame True {
                  n482 = local read "HASO ready"() -> (w1489:bool)
                  n483 = case shown="True" w1489 {
                    tunnel: w1498 -> [_ w1528]
                    tunnel: w1496 -> [_ w1527]
                    tunnel: w1495 -> [_ w1526]
                    tunnel: [w1499 w1523] -> w1487
                    tunnel: w1497 -> [_ w1521]
                    tunnel: [w1504 w1520] -> _
                    tunnel: w1490 -> [w1504 w1505]
                    tunnel: w1488 -> [w1499 w1506]
                    tunnel: w1493 -> [w1502 w1508]
                    tunnel: w1492 -> [w1501 w1519]
                    tunnel: [w1502 w1510] -> w1486
                    tunnel: [w1501 w1518] -> _
                    tunnel: w1494 -> [w1503 w1517]
                    tunnel: w1491 -> [w1500 w1516]
                    tunnel: [w1503 w1515] -> _
                    tunnel: [w1500 w1514] -> _
                    frame False {
                    }
                    frame True {
                      n484 = property on="nb_images (set)" class="DigNum (strict)"() -> ("Value"=w1529:u32)  [unwired: 2 in, 2 out]
                      n485 = case shown="2, Default" w1529 {
                        tunnel: [w1609 w1611] -> w1530
                        tunnel: w1521 -> [w1608 _]
                        tunnel: w1528 -> [w1609 _]
                        tunnel: [w1608 w1610] -> w1525
                        tunnel: w1527 -> [_ w1611]
                        tunnel: w1526 -> [_ w1610]
                        frame 2, Default {
                        }
                        frame 1 {
                        }
                      }
                      n486 = call <userlib>:"LVClass_Camera get image.vi"("Camera in"=w1505, "Image"=w1530, "Image RAW"=w1525, "remove_background"=FALSE, "error in (no error)"=w1506) -> ("Camera out"=w1520:refnum<class "Camera.lvclass">, "Image (dup)"=w1524:refnum<class "Image.lvclass">, "error out"=w1522:errorcluster)  [unwired: 7 in, 1 out]
                      n487 = case shown="No Error" w1522 {
                        selector: w1522 -> [w1605 w1606]
                        tunnel: w1524 -> [w1602 w1607]
                        tunnel: [w1601 w1607] -> w1513
                        tunnel: [w1600 w1606] -> w1512
                        frame No Error {
                          # "get image"
                          n488 = call <userlib>:"LVClass_Image get image data.vi"("Image in"=w1602, "error in (no error)"=w1605) -> ("Image out"=w1604:refnum<class "Image.lvclass">, "Image data out"=w1599:u32[][], "error out"=w1603:errorcluster)  [unwired: 11 in]
                          n489 = call <userlib>:"LVClass_Image get image information.vi"("Image in"=w1604, "error in (no error)"=w1603) -> ("Image out"=w1601:refnum<class "Image.lvclass">, "error out"=w1600:errorcluster)  [unwired: 11 in, 1 out]
                          n490 = local write "HASO intensity"(w1599) -> ()
                        }
                        frame Error {
                        }
                      }
                      n491 = case shown="No Error" w1512 {
                        selector: w1512 -> [w1557 w1598]
                        tunnel: [w1563 w1598] -> w1523
                        tunnel: w1513 -> [w1556 _]
                        tunnel: [w1561 w1595] -> w1514
                        tunnel: [w1560 w1597] -> w1515
                        tunnel: refnum<class "HasoSlopes.lvclass"> refnum ("HasoSlopes in") -> [w1553 w1594]
                        tunnel: w1519 -> [w1552 w1596]
                        tunnel: [w1551 w1596] -> w1518
                        tunnel: w1517 -> [w1550 w1597]
                        tunnel: w1516 -> [w1548 w1595]
                        tunnel: [w1533 w1593] -> w1510
                        tunnel: [w1531 w1594] -> w1509
                        tunnel: w1508 -> [w1532 w1593]
                        frame No Error {
                          # "phaseout"
                          n492 = local read "File Base Name"() -> (w1540:string)
                          n493 = local read "Save File"() -> (w1541:bool)
                          n494 = local read "Output path"() -> (w1539:path)
                          n495 = call "image2slopes.vi"("error in (no error)"=w1557, "Image in"=w1556, "HasoEngine in"=w1552, "HasoSlopes in"=w1553) -> ("error out"=w1535:errorcluster, "HasoEngine out"=w1551:refnum<class "HasoEngine.lvclass">, "HasoSlopes out"=w1531:refnum<class "HasoSlopes.lvclass">)  [unwired: 4 in, 1 out]
                          n496 = local read "Filter"() -> (w1547:u8[])
                          n497 = call <userlib>:"LVClass_HasoSlopes Apply Substractor.vi"("HasoSlopes in"=w1532, "HasoSlopes to substract"=w1531, "error in (no error)"=w1535) -> ("HasoSlopes out"=w1536:refnum<class "HasoSlopes.lvclass">, "error out"=w1534:errorcluster)  [unwired: 11 in]
                          n498 = call "slopes2phase.vi"("TypePhase"=WavefrontReconstructionMode."Modal_Zernike", "Number of coefficients"=u8 32, "error in (no error)"=w1534, "Filter"=w1547, "HasoSlopes in"=w1536, "Phase in"=w1550) -> ("error out"=w1543:errorcluster, "HasoSlopes out"=w1544:refnum<class "HasoSlopes.lvclass">, "Phase out"=w1549:refnum<class "Phase.lvclass">)  [unwired: 3 in]
                          n499 = local read "idxType"() -> (w1538:enum16{"Wyant", "ANSI"})
                          n500 = call "slopes2zern.vi"("HasoSlopes in"=w1544, "error in (no error)"=w1543, "idxType"=w1538) -> ("HasoSlopes out"=w1533:refnum<class "HasoSlopes.lvclass">, "Zernike Coefficients"=w1537:dbl[], "error out"=w1542:errorcluster)  [unwired: 3 in, 2 out]
                          n501 = call <userlib>:"LVClass_Pupil ctor from HasoSlopes.vi"("Pupil in"=w1548, "HasoSlopes.lvclass"=w1536, "error in (no error)"=w1542) -> ("Pupil out"=w1558:refnum<class "Pupil.lvclass">, "error out"=w1559:errorcluster)  [unwired: 11 in]
                          n502 = case shown="True" w1541 {
                            tunnel: w1540 -> [_ w1569]
                            tunnel: w1539 -> [_ w1568]
                            tunnel: w1537 -> [_ w1567]
                            tunnel: w1536 -> [_ w1565]
                            tunnel: w1531 -> [_ w1566]
                            frame False {
                            }
                            frame True {
                              n503 = stacked-sequence {
                                tunnel: w1569 -> [w1573 w1580 w1586]
                                tunnel: w1568 -> [w1572 w1579 w1585]
                                tunnel: w1567 -> [_ _ w1584]
                                tunnel: w1566 -> [w1570 _ _]
                                tunnel: w1565 -> [_ w1577 _]
                                frame #0 {
                                n504 = Concatenate Strings(w1573, "_slopesOffset", ".has") -> (w1576:string)
                                n505 = Build Path(base path=w1572, name or relative path=w1576) -> (appended path=w1571:path)
                                n506 = call <userlib>:"LVClass_HasoSlopes Save.vi"("HasoSlopes in"=w1570, "path"=w1571) -> ()  [unwired: 12 in, 2 out]
                                }
                                frame #1 {
                                n507 = Concatenate Strings(w1580, "_slopesNet", ".has") -> (w1583:string)
                                n508 = Build Path(base path=w1579, name or relative path=w1583) -> (appended path=w1578:path)
                                n509 = call <userlib>:"LVClass_HasoSlopes Save.vi"("HasoSlopes in"=w1577, "path"=w1578) -> ()  [unwired: 12 in, 2 out]
                                }
                                frame #2 {
                                n510 = Concatenate Strings(w1586, "_zernCoefNet", ".txt") -> (w1589:string)
                                n511 = Build Path(base path=w1585, name or relative path=w1589) -> (appended path=w1590:path)
                                n512 = Array To Spreadsheet String(array=w1584, 3:"%f") -> (spreadsheet string=w1591:string)  [unwired: 1 in]
                                n513 = Write to Text File(file (use dialog)=w1590, text=w1591) -> ()  [unwired: 2 in, 3 out]
                                }
                              }
                            }
                          }
                          n514 = call <userlib>:"LVClasse_Phase GetStatisticDatas.vi"("Phase in"=w1549, "error in (no error)"=w1559) -> ("Phase out"=w1564:refnum<class "Phase.lvclass">, "StatisticsData"=w1545:T2, "error out"=w1562:errorcluster)  [unwired: 11 in]
                          n515 = local write "Phase statistics"(w1545) -> ()
                          n516 = call <userlib>:"LVClasse_Phase Get Data.vi"("Phase in"=w1564, "Pupil"=w1558, "error in (no error)"=w1562) -> ("Phase out"=w1560:refnum<class "Phase.lvclass">, "data"=w1546:sgl[][], "Pupil (dup)"=w1561:refnum<class "Pupil.lvclass">, "error out"=w1563:errorcluster)  [unwired: 9 in]
                          n517 = local write "Zernike Measured"(w1537) -> ()
                          n518 = local write "Phase values"(w1546) -> ()
                        }
                        frame Error {
                        }
                      }
                      n519 = call <userlib>:"LVClass_HasoSlopes dtor.vi"("HasoSlopes in"=w1509) -> ()  [unwired: 13 in, 2 out]
                    }
                  }
                }
              }
              n520 = Unbundle By Name(w1473) -> ("status"=w1474:bool)
            }
          }
        }
      }
      event "Exit": Value Change {
        # "STOP AND EXIT"
        n521 = event-data() -> ()  [unwired: 1 in, 4 out]
        n522 = case shown="False" w1617 {
          tunnel: w1625 -> [w1628 w1631]
          tunnel: [errorcluster {"status"=FALSE, "code"=0, "source"=""} ("error out") w1630] -> w1624
          tunnel: [w1628 w1629] -> w1623
          frame False {
          }
          frame True {
            n523 = call <userlib>:"LVClass_Camera stop acquisition.vi"("Camera in"=w1631) -> ("Camera out"=w1629:refnum<class "Camera.lvclass">, "error out"=w1630:errorcluster)  [unwired: 13 in]
          }
        }
      }
      event Panel Close? {
        n524 = event-data() -> ()  [unwired: 1 in, 1 out]
        n525 = flat-sequence {
          tunnel: w1647 -> [w1653]
          tunnel: w1640 -> [w1650]
          tunnel: [w1652] -> w1633
          tunnel: [w1651] -> w1632
          tunnel: [w1655] -> w1645
          tunnel: [w1656] -> w1646
          tunnel: w1633 -> [w1656]
          tunnel: w1632 -> [w1655]
          frame #0 {
            n526 = call <userlib>:"LVClass_Camera stop acquisition.vi"("Camera in"=w1653, "error in (no error)"=w1650) -> ("Camera out"=w1652:refnum<class "Camera.lvclass">, "error out"=w1651:errorcluster)  [unwired: 12 in]
          }
          frame #1 {
            n527 = local write "HASO ready"(FALSE) -> ()
          }
        }
        n528 = event-data("Discard?"=TRUE) -> ()  [unwired: 1 in, 1 out]
      }
    }
    n529 = Wait (ms)(milliseconds to wait=u32 250) -> ()  [unwired: 1 out]
  }
  n530 = case shown="True" w24 {
    tunnel: w46 -> [_ w1681]
    tunnel: w45 -> [_ w1680]
    tunnel: w44 -> [_ w1679]
    tunnel: w43 -> [_ w1678]
    tunnel: w42 -> [_ w1677]
    tunnel: w41 -> [_ w1676]
    tunnel: w40 -> [_ w1675]
    tunnel: w9 -> [_ w1668]
    tunnel: w5 -> [_ w1667]
    tunnel: w4 -> [_ w1666]
    tunnel: w3 -> [_ w1665]
    tunnel: w1 -> [_ w1662]
    tunnel: w2 -> [_ w1657]
    frame False {
    }
    frame True {
      n531 = flat-sequence {
        tunnel: w1680 -> [w1718]
        tunnel: w1681 -> [w1716]
        tunnel: [w1718] -> w1695
        tunnel: w1675 -> [w1717]
        tunnel: [w1717] -> w1694
        tunnel: [w1716] -> w1693
        tunnel: w1679 -> [w1715]
        tunnel: w1678 -> [w1714]
        tunnel: w1677 -> [w1713]
        tunnel: w1676 -> [w1712]
        tunnel: [w1711] -> w1692
        tunnel: [w1710] -> w1691
        tunnel: [w1709] -> w1690
        tunnel: [w1708] -> w1689
        tunnel: [w1701] -> w1673
        tunnel: [w1702] -> w1671
        tunnel: [w1703] -> w1669
        tunnel: w1668 -> [w1707]
        tunnel: w1667 -> [w1706]
        tunnel: w1666 -> [w1705]
        tunnel: w1665 -> [w1704]
        tunnel: [w1700] -> w1663
        tunnel: w1662 -> [w1699]
        tunnel: [w1698] -> w1661
        tunnel: w1657 -> [w1697]
        tunnel: [w1697] -> w1658
        tunnel: w1695 -> [w1733]
        tunnel: w1694 -> [w1732]
        tunnel: w1693 -> [w1730]
        tunnel: [w1732] -> w1688
        tunnel: [w1731] -> w1687
        tunnel: [w1730] -> w1686
        tunnel: w1692 -> [w1729]
        tunnel: [w1729] -> w1685
        tunnel: w1691 -> [w1728]
        tunnel: [w1728] -> w1684
        tunnel: w1690 -> [w1727]
        tunnel: [w1727] -> w1683
        tunnel: w1689 -> [w1726]
        tunnel: [w1726] -> w1682
        tunnel: [w1725] -> w1674
        tunnel: w1673 -> [w1725]
        tunnel: [w1724] -> w1672
        tunnel: w1671 -> [w1724]
        tunnel: [w1723] -> w1670
        tunnel: w1669 -> [w1723]
        tunnel: [w1722] -> w1664
        tunnel: w1663 -> [w1722]
        tunnel: w1661 -> [w1721]
        tunnel: [w1721] -> w1660
        tunnel: [w1720] -> w1659
        tunnel: w1658 -> [w1719]
        tunnel: w1688 -> [w1749]
        tunnel: w1687 -> [w1747]
        tunnel: w1686 -> [w1746]
        tunnel: w1685 -> [w1745]
        tunnel: w1684 -> [w1744]
        tunnel: w1683 -> [w1743]
        tunnel: w1682 -> [w1742]
        tunnel: w1674 -> [w1740]
        tunnel: w1672 -> [w1739]
        tunnel: w1670 -> [w1738]
        tunnel: w1664 -> [w1737]
        tunnel: w1660 -> [w1736]
        tunnel: w1659 -> [w1735]
        frame #0 {
          n532 = call <userlib>:"LVClass_Image dtor.vi"("Image in"=w1714) -> ("error out"=w1710:errorcluster)  [unwired: 13 in, 1 out]
          n533 = local write "HASO ready"(FALSE) -> ()
          n534 = call <userlib>:"LVClass_HasoSlopes dtor.vi"("HasoSlopes in"=w1707) -> ("error out"=w1702:errorcluster)  [unwired: 13 in, 1 out]
          n535 = call <userlib>:"LVClass_Pupil dtor.vi"("Pupil in"=w1704) -> ("error out"=w1700:errorcluster)  [unwired: 13 in, 1 out]
          n536 = call <userlib>:"LVClass_Image dtor.vi"("Image in"=w1712) -> ("error out"=w1708:errorcluster)  [unwired: 13 in, 1 out]
          n537 = call <userlib>:"LVClass_WavefrontCorrector dtor.vi"("WavefrontCorrector in"=w1699) -> ("error out"=w1698:errorcluster)  [unwired: 13 in, 1 out]
          n538 = call <userlib>:"LVClass_Image dtor.vi"("Image in"=w1715) -> ("error out"=w1711:errorcluster)  [unwired: 13 in, 1 out]
          n539 = call <userlib>:"LVClass_Image dtor.vi"("Image in"=w1713) -> ("error out"=w1709:errorcluster)  [unwired: 13 in, 1 out]
          n540 = call <userlib>:"LVClass_HasoEngine dtor.vi"("HasoEngine in"=w1705) -> ("error out"=w1701:errorcluster)  [unwired: 13 in, 1 out]
          n541 = call <userlib>:"LVClasse_Phase dtor.vi"("Phase in"=w1706) -> ("error out"=w1703:errorcluster)  [unwired: 13 in, 1 out]
        }
        frame #1 {
          n542 = call <userlib>:"LVClass_Camera dtor.vi"("Camera in"=w1733) -> ("error out"=w1731:errorcluster)  [unwired: 13 in, 1 out]
          n543 = call <userlib>:"LVClass_WavefrontCorrectorSet dtor.vi"("WavefrontCorrectorSet in"=w1719) -> ("error out"=w1720:errorcluster)  [unwired: 13 in, 1 out]
        }
        frame #2 {
          n544 = call <userlib>:"LVClass_CameraSet dtor.vi"("CameraSet.lvclass"=w1749) -> ("error out"=w1748:errorcluster)  [unwired: 13 in, 1 out]
          n545 = local write "Current status"("Shut down") -> ()
          n546 = Merge Errors(w1748, w1747, w1746, w1745, w1744, w1743, w1742, w1738, w1739, w1740, w1737, w1736, w1735) -> (w1741:errorcluster)
          n547 = property on="Current error" class="Clust (strict)"("Value"=w1741) -> ()  [unwired: 2 in, 2 out]
        }
      }
    }
  }
